vi "BRig_RT__Case_Exp__State_initTrial__LC_Cue__v18.vi"(6 "input_arrTrig":bool[](array[boolean]), 8 "input_dataTrial":u16[][](array[numeric]), 9 "input_dataExp":u16[](array[numeric]), 10 "input_dataLC":u16[](array[numeric]), 11 "input_dataCurrent":u16[](array[numeric])) -> (0 "output_dataTrial":u16[][](array[numeric]), 3 "output_dataCurrent":u16[](array[numeric]), 4 "output_arrTrig":bool[](array[boolean]))   [LabVIEW 2014]
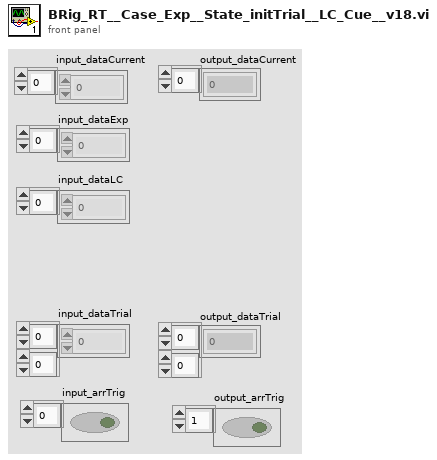
[diagram p1: front panel]
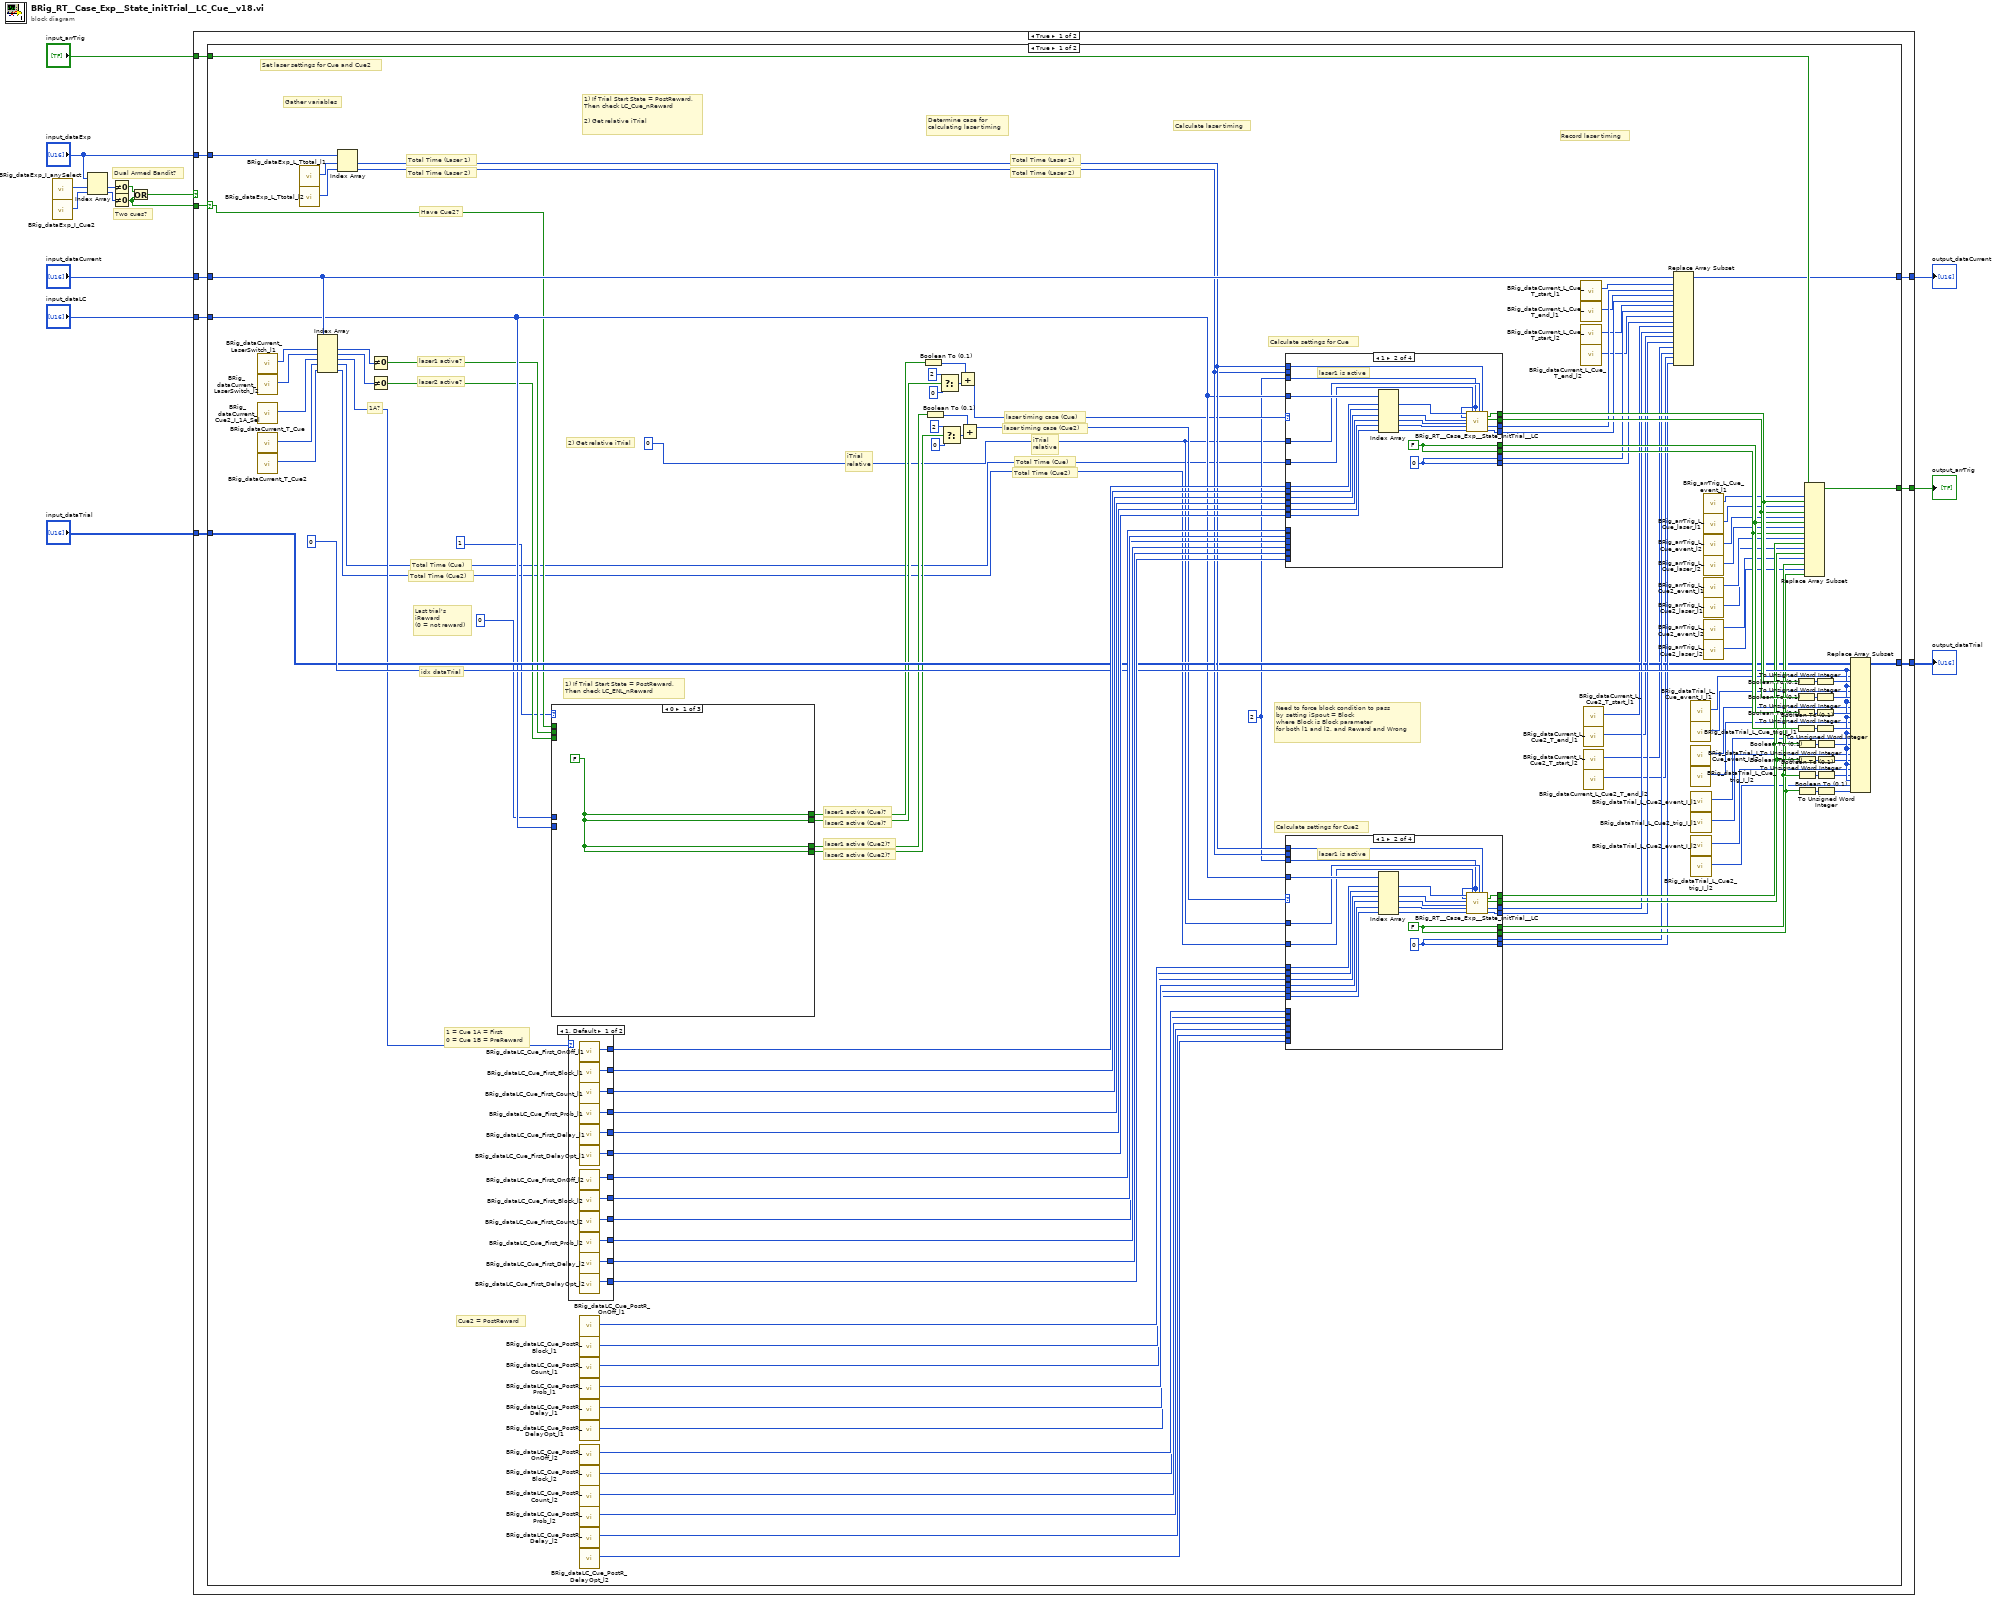
[diagram p0: block diagram]
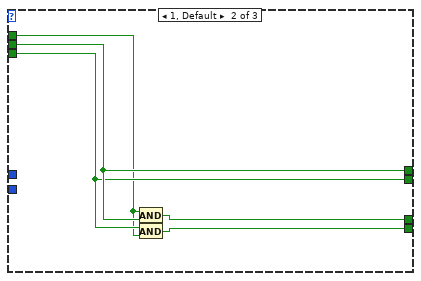
[diagram p2: hidden frame]
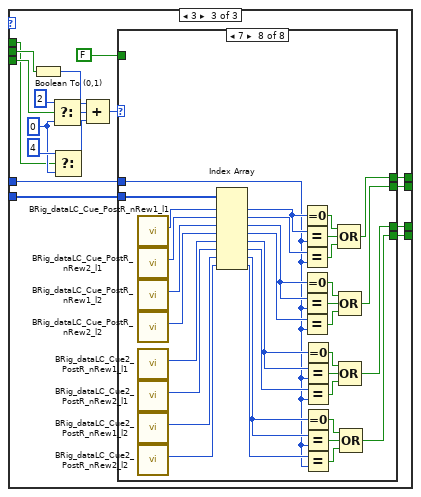
[diagram p3: hidden frame]
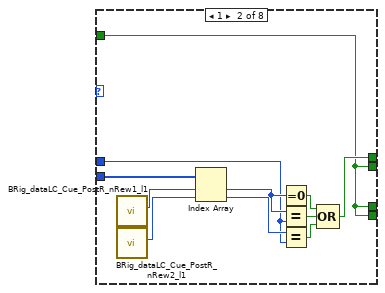
[diagram p5: hidden frame]
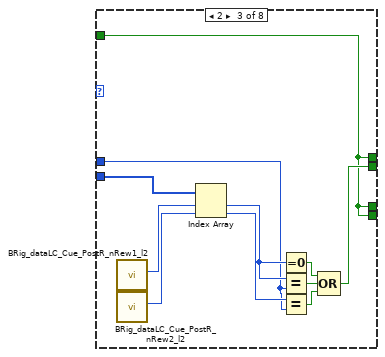
[diagram p6: hidden frame]
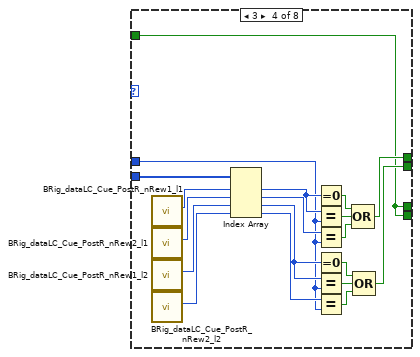
[diagram p7: hidden frame]
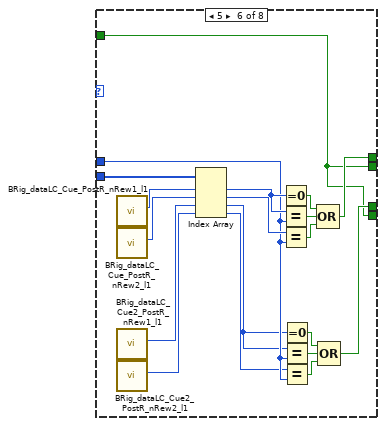
[diagram p9: hidden frame]
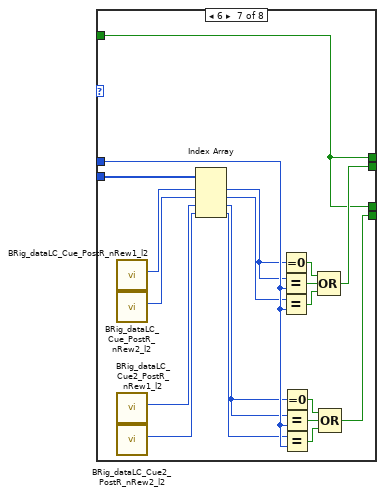
[diagram p10: hidden frame]
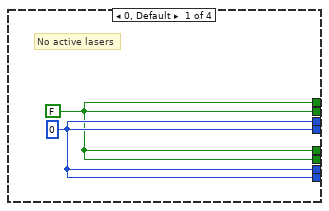
[diagram p11: hidden frame]
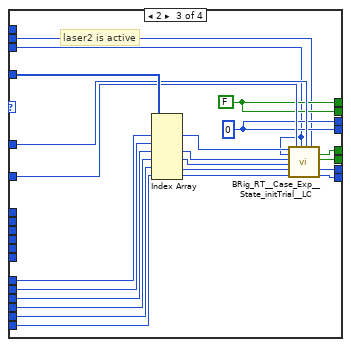
[diagram p12: hidden frame]
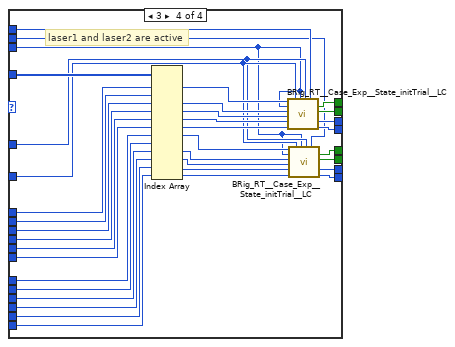
[diagram p13: hidden frame]
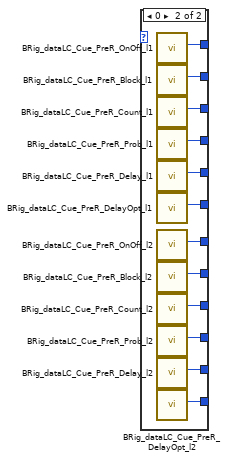
[diagram p14: hidden frame]
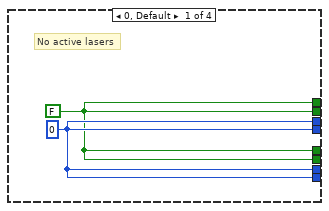
[diagram p15: hidden frame]
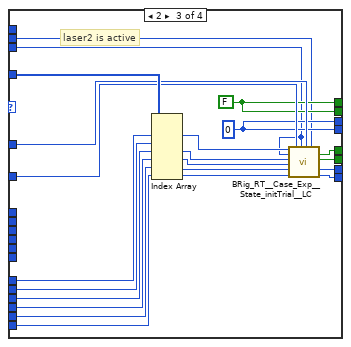
[diagram p16: hidden frame]
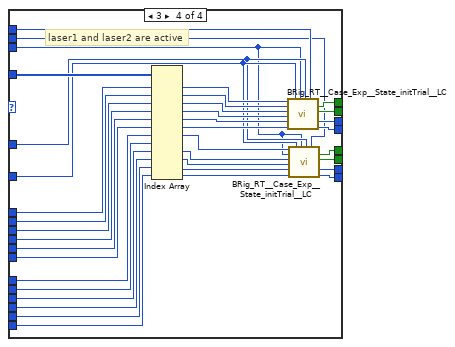
[diagram p17: hidden frame]
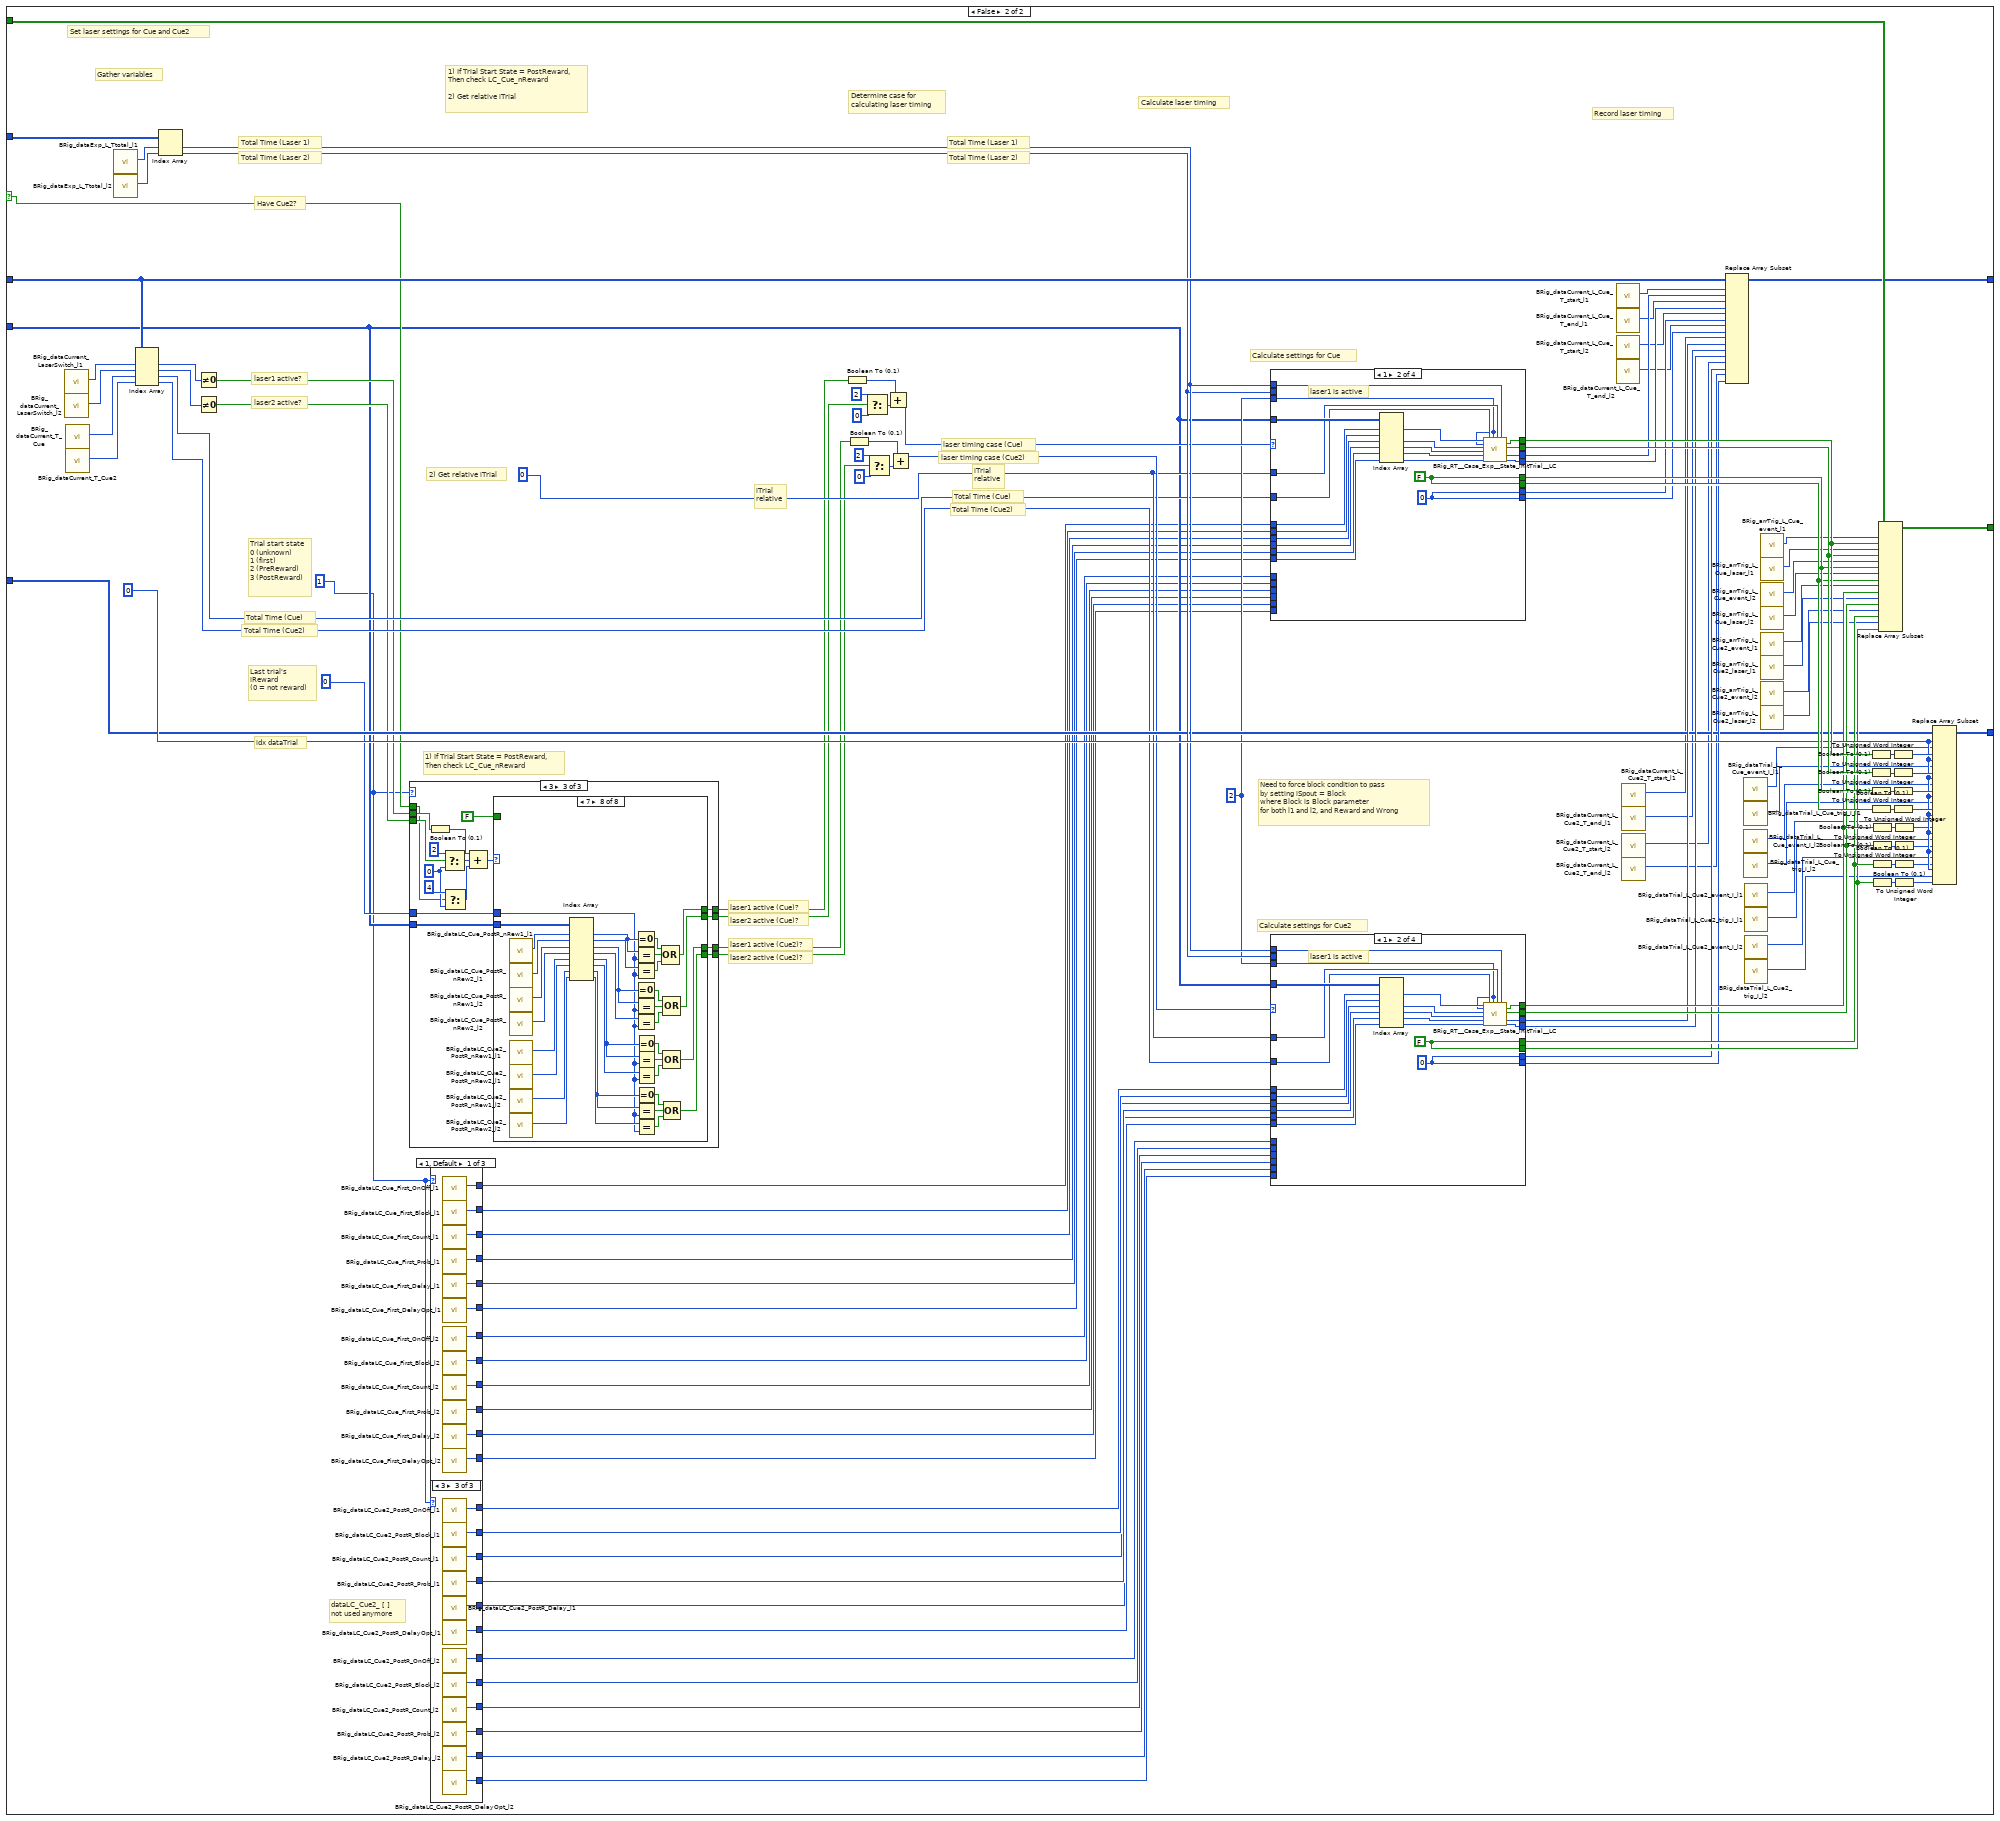
[diagram p18: hidden frame]
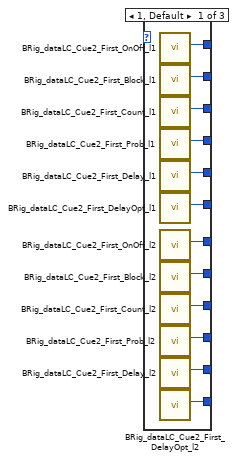
[diagram p19: hidden frame]
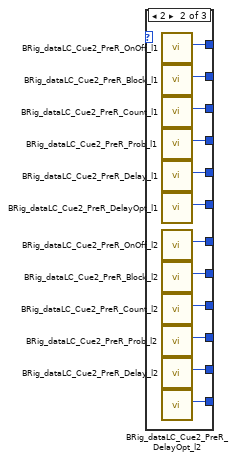
[diagram p20: hidden frame]
diagram:
  # "Two cues?"
  # "Dual Armed Bandit?"
  n1 = call "BRig_dataExp_I_anySelect.vi"() -> ("output_I_anySelect"=w8:i32)  [unwired: 11 in]
  n2 = call "BRig_dataExp_I_Cue2.vi"() -> ("output_I_Cue2"=w6:i32)  [unwired: 11 in]
  n3 = Index Array(array="input_dataExp", index #1=w8, index #2=w6) -> (element #1=w7:u16, element #2=w5:u16)
  n4 = Not Equal To 0?(x=w7) -> (x != 0?=w4:bool)
  n5 = Not Equal To 0?(x=w5) -> (x != 0?=w1:bool)
  n6 = Or(x=w4, y=w1) -> (x .or. y?=w2:bool)
  n7 = case shown="True" w2 {
    tunnel: "input_arrTrig" -> [w24 w1044]
    tunnel: [w23 w1043] -> w14
    tunnel: [w22 w1030] -> w13
    tunnel: "input_dataCurrent" -> [w21 w1029]
    tunnel: [w20 w1028] -> w11
    tunnel: "input_dataExp" -> [w19 w1021]
    tunnel: "input_dataTrial" -> [w18 w1012]
    tunnel: "input_dataLC" -> [w17 w1000]
    tunnel: w1 -> [w16 _]
    frame True {
      n8 = case shown="True" w16 {
        selector: w16 -> [w69 w533]
        tunnel: w24 -> [w140 w589]
        tunnel: [w139 w588] -> w23
        tunnel: [w126 w575] -> w22
        tunnel: w21 -> [w125 w574]
        tunnel: [w124 w573] -> w20
        tunnel: w19 -> [w105 w566]
        tunnel: w18 -> [w85 w546]
        tunnel: w17 -> [w84 w529]
        frame True {
          w70 = u16 0
          w71 = u16 2 ("input_sState_start")
          w100 = 0
          # "Cue2 = PostReward"
          # "1 = Cue 1A = First\n0 = Cue 1B = PreReward"
          # "1A?"
          # "Need to force block condition to pass\nby setting iSpout = Block\nwhere Block is Block parameter\nfor both l1 and l2, and Reward and Wrong"
          # "Record laser timing"
          # "Calculate laser timing"
          # "Total Time (Cue2)"
          # "Total Time (Cue)"
          # "iTrial\nrelative"
          # "Total Time (Laser 2)"
          # "Total Time (Laser 1)"
          # "laser timing case (Cue2)"
          # "Determine case for\ncalculating laser timing"
          # "2) Get relative iTrial"
          # "1) If Trial Start State = PostReward,\nThen check LC_ENL_nReward"
          # "laser2 active (Cue2)?"
          # "laser1 active (Cue2)?"
          # "laser2 active (Cue)?"
          # "laser1 active (Cue)?"
          # "1) If Trial Start State = PostReward,\nThen check LC_Cue_nReward\n\n2) Get relative iTrial"
          # "Gather variables"
          # "Last trial's\niReward\n(0 = not reward)"
          # "idx dataTrial"
          # "Total Time (Cue2)"
          # "Total Time (Cue)"
          # "Have Cue2?"
          # "Total Time (Laser 2)"
          # "Total Time (Laser 1)"
          # "Calculate settings for Cue2"
          # "Calculate settings for Cue"
          # "Set laser settings for Cue and Cue2"
          # "iTrial\nrelative"
          # "laser timing case (Cue)"
          # "laser2 active?"
          # "laser1 active?"
          n9 = call "BRig_dataCurrent_LaserSwitch_l1.vi"() -> ("output_LaserSwitch_l1"=w148:i32)  [unwired: 11 in]
          n10 = call "BRig_dataCurrent_LaserSwitch_l2.vi"() -> ("output_LaserSwitch_l2"=w147:i32)  [unwired: 11 in]
          n11 = call "BRig_dataCurrent_Cue2_I_1A_Sel.vi"() -> ("output_Cue2_I_1A_Sel"=w67:i32)  [unwired: 11 in]
          n12 = call "BRig_dataCurrent_T_Cue.vi"() -> ("output_T_Cue"=w64:i32)  [unwired: 11 in]
          n13 = call "BRig_dataCurrent_T_Cue2.vi"() -> ("output_T_Cue2"=w63:i32)  [unwired: 11 in]
          n14 = call "BRig_dataExp_L_Ttotal_l1.vi"() -> ("output_L_Ttotal_l1"=w106:i32)  [unwired: 11 in]
          n15 = call "BRig_dataExp_L_Ttotal_l2.vi"() -> ("output_L_Ttotal_l2"=w107:i32)  [unwired: 11 in]
          n16 = Index Array(array=w125, index #1=w148, index #2=w147, index #3=w67, index #4=w64, index #5=w63) -> (element #1=w146:u16, element #2=w145:u16, element #3=w66:u16, element #4=w61:u16, element #5=w62:u16)
          n17 = Index Array(array=w105, index #1=w106, index #2=w107) -> (element #1=w95:u16, element #2=w94:u16)
          n18 = Not Equal To 0?(x=w146) -> (x != 0?=w82:bool)
          n19 = Not Equal To 0?(x=w145) -> (x != 0?=w83:bool)
          n20 = case shown="0" u16 1 {
            tunnel: u16 0 -> [_ _ w162]
            tunnel: w84 -> [_ _ w161]
            tunnel: w83 -> [_ w153 w164]
            tunnel: w82 -> [_ w154 w165]
            tunnel: w69 -> [_ w152 w163]
            tunnel: [w149 w154 w158] -> w81
            tunnel: [w149 w153 w157] -> w80
            tunnel: [w149 w151 w156] -> w75
            tunnel: [w149 w150 w155] -> w74
            frame 0 {
              w149 = FALSE
            }
            frame 1, Default {
              n21 = And(x=w152, y=w154) -> (x .and. y?=w151:bool)
              n22 = And(x=w153, y=w152) -> (x .and. y?=w150:bool)
            }
            frame 3 {
              w169 = i16 0 ("f")
              n23 = Boolean To (0,1)(Boolean=w165) -> (0, 1=w167:i16)
              n24 = Select(t=i16 2, s=w164, f=w169) -> (s? t:f=w168:i16)
              n25 = Select(t=i16 4, s=w163, f=w169) -> (s? t:f=w166:i16)
              n26 = Compound Arithmetic op=ADD(w167, w168, w166) -> (w159:i16)
              n27 = case shown="7" w159 {
                tunnel: w161 -> [_ w178 w189 w203 _ w228 w249 w276]
                tunnel: w162 -> [_ w177 w188 w202 _ w224 w245 w265]
                tunnel: [w172 w176 w186 w201 w214 w223 w242 w264] -> w158
                tunnel: [w172 w175 w187 w200 w214 w221 w244 w263] -> w157
                tunnel: [w172 w175 w186 w199 w214 w222 w242 w262] -> w156
                tunnel: [w172 w175 w186 w199 w214 w221 w243 w261] -> w155
                tunnel: FALSE -> [w172 w175 w186 w199 w214 w221 w242 _]
                frame 0, Default {
                }
                frame 1 {
                  n28 = call "BRig_dataLC_Cue_PostR_nRew1_l1.vi"() -> ("output_Cue_PostR_nRew1_l1"=w173:i32)  [unwired: 11 in]
                  n29 = call "BRig_dataLC_Cue_PostR_nRew2_l1.vi"() -> ("output_Cue_PostR_nRew2_l1"=w174:i32)  [unwired: 11 in]
                  n30 = Index Array(array=w178, index #1=w173, index #2=w174) -> (element #1=w180:u16, element #2=w179:u16)
                  n31 = Equal To 0?(x=w180) -> (x = 0?=w181:bool)
                  n32 = Equal?(x=w180, y=w177) -> (x = y?=w182:bool)
                  n33 = Equal?(x=w179, y=w177) -> (x = y?=w183:bool)
                  n34 = Compound Arithmetic op=OR(w181, w182, w183) -> (w176:bool)
                }
                frame 2 {
                  n35 = call "BRig_dataLC_Cue_PostR_nRew1_l2.vi"() -> ("output_Cue_PostR_nRew1_l2"=w184:i32)  [unwired: 11 in]
                  n36 = call "BRig_dataLC_Cue_PostR_nRew2_l2.vi"() -> ("output_Cue_PostR_nRew2_l2"=w185:i32)  [unwired: 11 in]
                  n37 = Index Array(array=w189, index #1=w184, index #2=w185) -> (element #1=w190:u16, element #2=w191:u16)
                  n38 = Equal To 0?(x=w190) -> (x = 0?=w193:bool)
                  n39 = Equal?(x=w190, y=w188) -> (x = y?=w192:bool)
                  n40 = Equal?(x=w191, y=w188) -> (x = y?=w194:bool)
                  n41 = Compound Arithmetic op=OR(w193, w192, w194) -> (w187:bool)
                }
                frame 3 {
                  n42 = call "BRig_dataLC_Cue_PostR_nRew1_l1.vi"() -> ("output_Cue_PostR_nRew1_l1"=w195:i32)  [unwired: 11 in]
                  n43 = call "BRig_dataLC_Cue_PostR_nRew2_l1.vi"() -> ("output_Cue_PostR_nRew2_l1"=w196:i32)  [unwired: 11 in]
                  n44 = call "BRig_dataLC_Cue_PostR_nRew1_l2.vi"() -> ("output_Cue_PostR_nRew1_l2"=w197:i32)  [unwired: 11 in]
                  n45 = call "BRig_dataLC_Cue_PostR_nRew2_l2.vi"() -> ("output_Cue_PostR_nRew2_l2"=w198:i32)  [unwired: 11 in]
                  n46 = Index Array(array=w203, index #1=w195, index #2=w196, index #3=w197, index #4=w198) -> (element #1=w207:u16, element #2=w206:u16, element #3=w204:u16, element #4=w205:u16)
                  n47 = Equal To 0?(x=w207) -> (x = 0?=w208:bool)
                  n48 = Equal?(x=w207, y=w202) -> (x = y?=w209:bool)
                  n49 = Equal?(x=w206, y=w202) -> (x = y?=w210:bool)
                  n50 = Equal To 0?(x=w204) -> (x = 0?=w212:bool)
                  n51 = Equal?(x=w204, y=w202) -> (x = y?=w211:bool)
                  n52 = Equal?(x=w205, y=w202) -> (x = y?=w213:bool)
                  n53 = Compound Arithmetic op=OR(w208, w209, w210) -> (w201:bool)
                  n54 = Compound Arithmetic op=OR(w212, w211, w213) -> (w200:bool)
                }
                frame 4 {
                }
                frame 5 {
                  n55 = call "BRig_dataLC_Cue_PostR_nRew1_l1.vi"() -> ("output_Cue_PostR_nRew1_l1"=w217:i32)  [unwired: 11 in]
                  n56 = call "BRig_dataLC_Cue_PostR_nRew2_l1.vi"() -> ("output_Cue_PostR_nRew2_l1"=w218:i32)  [unwired: 11 in]
                  n57 = call "BRig_dataLC_Cue2_PostR_nRew1_l1.vi"() -> ("output_Cue2_PostR_nRew1_l1"=w215:i32)  [unwired: 11 in]
                  n58 = call "BRig_dataLC_Cue2_PostR_nRew2_l1.vi"() -> ("output_Cue2_PostR_nRew2_l1"=w216:i32)  [unwired: 11 in]
                  n59 = Index Array(array=w228, index #1=w217, index #2=w218, index #3=w215, index #4=w216) -> (element #1=w230:u16, element #2=w229:u16, element #3=w220:u16, element #4=w219:u16)
                  n60 = Equal To 0?(x=w230) -> (x = 0?=w231:bool)
                  n61 = Equal?(x=w230, y=w224) -> (x = y?=w232:bool)
                  n62 = Equal?(x=w229, y=w224) -> (x = y?=w233:bool)
                  n63 = Equal To 0?(x=w220) -> (x = 0?=w227:bool)
                  n64 = Equal?(x=w220, y=w224) -> (x = y?=w226:bool)
                  n65 = Equal?(x=w219, y=w224) -> (x = y?=w225:bool)
                  n66 = Compound Arithmetic op=OR(w231, w232, w233) -> (w223:bool)
                  n67 = Compound Arithmetic op=OR(w227, w226, w225) -> (w222:bool)
                }
                frame 6 {
                  n68 = call "BRig_dataLC_Cue_PostR_nRew1_l2.vi"() -> ("output_Cue_PostR_nRew1_l2"=w237:i32)  [unwired: 11 in]
                  n69 = call "BRig_dataLC_Cue_PostR_nRew2_l2.vi"() -> ("output_Cue_PostR_nRew2_l2"=w236:i32)  [unwired: 11 in]
                  n70 = call "BRig_dataLC_Cue2_PostR_nRew1_l2.vi"() -> ("output_Cue2_PostR_nRew1_l2"=w235:i32)  [unwired: 11 in]
                  n71 = call "BRig_dataLC_Cue2_PostR_nRew2_l2.vi"() -> ("output_Cue2_PostR_nRew2_l2"=w234:i32)  [unwired: 11 in]
                  n72 = Index Array(array=w249, index #1=w237, index #2=w236, index #3=w235, index #4=w234) -> (element #1=w241:u16, element #2=w240:u16, element #3=w239:u16, element #4=w238:u16)
                  n73 = Equal To 0?(x=w241) -> (x = 0?=w251:bool)
                  n74 = Equal?(x=w241, y=w245) -> (x = y?=w250:bool)
                  n75 = Equal?(x=w240, y=w245) -> (x = y?=w252:bool)
                  n76 = Equal To 0?(x=w239) -> (x = 0?=w247:bool)
                  n77 = Equal?(x=w239, y=w245) -> (x = y?=w248:bool)
                  n78 = Equal?(x=w238, y=w245) -> (x = y?=w246:bool)
                  n79 = Compound Arithmetic op=OR(w251, w250, w252) -> (w244:bool)
                  n80 = Compound Arithmetic op=OR(w247, w248, w246) -> (w243:bool)
                }
                frame 7 {
                  n81 = call "BRig_dataLC_Cue_PostR_nRew1_l1.vi"() -> ("output_Cue_PostR_nRew1_l1"=w257:i32)  [unwired: 11 in]
                  n82 = call "BRig_dataLC_Cue_PostR_nRew2_l1.vi"() -> ("output_Cue_PostR_nRew2_l1"=w258:i32)  [unwired: 11 in]
                  n83 = call "BRig_dataLC_Cue_PostR_nRew1_l2.vi"() -> ("output_Cue_PostR_nRew1_l2"=w259:i32)  [unwired: 11 in]
                  n84 = call "BRig_dataLC_Cue_PostR_nRew2_l2.vi"() -> ("output_Cue_PostR_nRew2_l2"=w260:i32)  [unwired: 11 in]
                  n85 = call "BRig_dataLC_Cue2_PostR_nRew1_l1.vi"() -> ("output_Cue2_PostR_nRew1_l1"=w256:i32)  [unwired: 11 in]
                  n86 = call "BRig_dataLC_Cue2_PostR_nRew2_l1.vi"() -> ("output_Cue2_PostR_nRew2_l1"=w255:i32)  [unwired: 11 in]
                  n87 = call "BRig_dataLC_Cue2_PostR_nRew1_l2.vi"() -> ("output_Cue2_PostR_nRew1_l2"=w254:i32)  [unwired: 11 in]
                  n88 = call "BRig_dataLC_Cue2_PostR_nRew2_l2.vi"() -> ("output_Cue2_PostR_nRew2_l2"=w253:i32)  [unwired: 11 in]
                  n89 = Index Array(array=w276, index #1=w257, index #2=w258, index #3=w259, index #4=w260, index #5=w256, index #6=w255, index #7=w254, index #8=w253) -> (element #1=w280:u16, element #2=w279:u16, element #3=w277:u16, element #4=w278:u16, element #5=w269:u16, element #6=w268:u16, element #7=w266:u16, element #8=w267:u16)
                  n90 = Equal To 0?(x=w280) -> (x = 0?=w281:bool)
                  n91 = Equal?(x=w280, y=w265) -> (x = y?=w282:bool)
                  n92 = Equal?(x=w279, y=w265) -> (x = y?=w283:bool)
                  n93 = Equal To 0?(x=w277) -> (x = 0?=w285:bool)
                  n94 = Equal?(x=w277, y=w265) -> (x = y?=w284:bool)
                  n95 = Equal?(x=w278, y=w265) -> (x = y?=w286:bool)
                  n96 = Equal To 0?(x=w269) -> (x = 0?=w275:bool)
                  n97 = Equal?(x=w269, y=w265) -> (x = y?=w274:bool)
                  n98 = Equal?(x=w268, y=w265) -> (x = y?=w273:bool)
                  n99 = Equal To 0?(x=w266) -> (x = 0?=w271:bool)
                  n100 = Equal?(x=w266, y=w265) -> (x = y?=w272:bool)
                  n101 = Equal?(x=w267, y=w265) -> (x = y?=w270:bool)
                  n102 = Compound Arithmetic op=OR(w281, w282, w283) -> (w264:bool)
                  n103 = Compound Arithmetic op=OR(w285, w284, w286) -> (w263:bool)
                  n104 = Compound Arithmetic op=OR(w275, w274, w273) -> (w262:bool)
                  n105 = Compound Arithmetic op=OR(w271, w272, w270) -> (w261:bool)
                }
              }
            }
          }
          n106 = case shown="1, Default" w66 {
            tunnel: [w370 w382] -> w119
            tunnel: [w371 w383] -> w118
            tunnel: [w372 w384] -> w117
            tunnel: [w373 w385] -> w116
            tunnel: [w374 w386] -> w115
            tunnel: [w375 w387] -> w114
            tunnel: [w376 w388] -> w113
            tunnel: [w377 w389] -> w112
            tunnel: [w378 w390] -> w111
            tunnel: [w379 w391] -> w110
            tunnel: [w380 w392] -> w109
            tunnel: [w369 w381] -> w108
            frame 1, Default {
              n107 = call "BRig_dataLC_Cue_First_OnOff_l1.vi"() -> ("output_Cue_First_OnOff"=w370:i32)  [unwired: 11 in]
              n108 = call "BRig_dataLC_Cue_First_Block_l1.vi"() -> ("output_Cue_First_Block"=w371:i32)  [unwired: 11 in]
              n109 = call "BRig_dataLC_Cue_First_Count_l1.vi"() -> ("output_Cue_First_Count"=w372:i32)  [unwired: 11 in]
              n110 = call "BRig_dataLC_Cue_First_Prob_l1.vi"() -> ("output_Cue_First_Prob"=w373:i32)  [unwired: 11 in]
              n111 = call "BRig_dataLC_Cue_First_Delay_l1.vi"() -> ("output_Cue_First_Delay"=w374:i32)  [unwired: 11 in]
              n112 = call "BRig_dataLC_Cue_First_DelayOpt_l1.vi"() -> ("output_Cue_First_DelayOpt"=w375:i32)  [unwired: 11 in]
              n113 = call "BRig_dataLC_Cue_First_OnOff_l2.vi"() -> ("output_Cue_First_OnOff_l2"=w376:i32)  [unwired: 11 in]
              n114 = call "BRig_dataLC_Cue_First_Block_l2.vi"() -> ("output_Cue_First_Block_l2"=w377:i32)  [unwired: 11 in]
              n115 = call "BRig_dataLC_Cue_First_Count_l2.vi"() -> ("output_Cue_First_Count_l2"=w378:i32)  [unwired: 11 in]
              n116 = call "BRig_dataLC_Cue_First_Prob_l2.vi"() -> ("output_Cue_First_Prob_l2"=w379:i32)  [unwired: 11 in]
              n117 = call "BRig_dataLC_Cue_First_Delay_l2.vi"() -> ("output_Cue_First_Delay_l2"=w380:i32)  [unwired: 11 in]
              n118 = call "BRig_dataLC_Cue_First_DelayOpt_l2.vi"() -> ("output_Cue_First_DelayOpt_l2"=w369:i32)  [unwired: 11 in]
            }
            frame 0 {
              n119 = call "BRig_dataLC_Cue_PreR_OnOff_l1.vi"() -> ("output_Cue_PreR_OnOff"=w382:i32)  [unwired: 11 in]
              n120 = call "BRig_dataLC_Cue_PreR_Block_l1.vi"() -> ("output_Cue_PreR_Block"=w383:i32)  [unwired: 11 in]
              n121 = call "BRig_dataLC_Cue_PreR_Count_l1.vi"() -> ("output_Cue_PreR_Count"=w384:i32)  [unwired: 11 in]
              n122 = call "BRig_dataLC_Cue_PreR_Prob_l1.vi"() -> ("output_Cue_PreR_Prob"=w385:i32)  [unwired: 11 in]
              n123 = call "BRig_dataLC_Cue_PreR_Delay_l1.vi"() -> ("output_Cue_PreR_Delay"=w386:i32)  [unwired: 11 in]
              n124 = call "BRig_dataLC_Cue_PreR_DelayOpt_l1.vi"() -> ("output_Cue_PreR_DelayOpt"=w387:i32)  [unwired: 11 in]
              n125 = call "BRig_dataLC_Cue_PreR_OnOff_l2.vi"() -> ("output_Cue_PreR_OnOff_l2"=w388:i32)  [unwired: 11 in]
              n126 = call "BRig_dataLC_Cue_PreR_Block_l2.vi"() -> ("output_Cue_PreR_Block_l2"=w389:i32)  [unwired: 11 in]
              n127 = call "BRig_dataLC_Cue_PreR_Count_l2.vi"() -> ("output_Cue_PreR_Count_l2"=w390:i32)  [unwired: 11 in]
              n128 = call "BRig_dataLC_Cue_PreR_Prob_l2.vi"() -> ("output_Cue_PreR_Prob_l2"=w391:i32)  [unwired: 11 in]
              n129 = call "BRig_dataLC_Cue_PreR_Delay_l2.vi"() -> ("output_Cue_PreR_Delay_l2"=w392:i32)  [unwired: 11 in]
              n130 = call "BRig_dataLC_Cue_PreR_DelayOpt_l2.vi"() -> ("output_Cue_PreR_DelayOpt_l2"=w381:i32)  [unwired: 11 in]
            }
          }
          n131 = call "BRig_dataLC_Cue_PostR_OnOff_l1.vi"() -> ("output_Cue_PostR_OnOff"=w60:i32)  [unwired: 11 in]
          n132 = call "BRig_dataLC_Cue_PostR_Block_l1.vi"() -> ("output_Cue_PostR_Block"=w59:i32)  [unwired: 11 in]
          n133 = call "BRig_dataLC_Cue_PostR_Count_l1.vi"() -> ("output_Cue_PostR_Count"=w58:i32)  [unwired: 11 in]
          n134 = call "BRig_dataLC_Cue_PostR_Prob_l1.vi"() -> ("output_Cue_PostR_Prob"=w57:i32)  [unwired: 11 in]
          n135 = call "BRig_dataLC_Cue_PostR_Delay_l1.vi"() -> ("output_Cue_PostR_Delay"=w56:i32)  [unwired: 11 in]
          n136 = call "BRig_dataLC_Cue_PostR_DelayOpt_l1.vi"() -> ("output_Cue_PostR_DelayOpt"=w55:i32)  [unwired: 11 in]
          n137 = call "BRig_dataLC_Cue_PostR_OnOff_l2.vi"() -> ("output_Cue_PostR_OnOff_l2"=w54:i32)  [unwired: 11 in]
          n138 = call "BRig_dataLC_Cue_PostR_Block_l2.vi"() -> ("output_Cue_PostR_Block_l2"=w53:i32)  [unwired: 11 in]
          n139 = call "BRig_dataLC_Cue_PostR_Count_l2.vi"() -> ("output_Cue_PostR_Count_l2"=w52:i32)  [unwired: 11 in]
          n140 = call "BRig_dataLC_Cue_PostR_Prob_l2.vi"() -> ("output_Cue_PostR_Prob_l2"=w51:i32)  [unwired: 11 in]
          n141 = call "BRig_dataLC_Cue_PostR_Delay_l2.vi"() -> ("output_Cue_PostR_Delay_l2"=w50:i32)  [unwired: 11 in]
          n142 = call "BRig_dataLC_Cue_PostR_DelayOpt_l2.vi"() -> ("output_Cue_PostR_DelayOpt_l2"=w49:i32)  [unwired: 11 in]
          n143 = Boolean To (0,1)(Boolean=w81) -> (0, 1=w142:i16)
          n144 = Boolean To (0,1)(Boolean=w75) -> (0, 1=w78:i16)
          n145 = Select(t=i16 2, s=w80, f=i16 0) -> (s? t:f=w143:i16)
          n146 = Select(t=i16 2, s=w74, f=i16 0) -> (s? t:f=w77:i16)
          n147 = Add(x=w142, y=w143) -> (x+y=w73:i16)
          n148 = Add(x=w78, y=w77) -> (x+y=w72:i16)
          n149 = case shown="1" w73 {
            tunnel: w84 -> [_ w416 w438 w475]
            tunnel: w71 -> [_ w395 w417 w439]
            tunnel: w61 -> [_ w410 w432 w463]
            tunnel: w70 -> [_ w409 w431 w462]
            tunnel: [w393 w408 w420 w461] -> w134
            tunnel: [w393 w407 w420 w460] -> w131
            tunnel: [w394 w406 w419 w459] -> w123
            tunnel: [w394 w405 w419 w458] -> w122
            tunnel: [w393 w398 w430 w457] -> w127
            tunnel: [w394 w397 w429 w456] -> w121
            tunnel: [w393 w398 w428 w455] -> w129
            tunnel: [w394 w397 w427 w454] -> w120
            tunnel: w119 -> [_ w404 _ w453]
            tunnel: w118 -> [_ w403 _ w452]
            tunnel: w117 -> [_ w402 _ w451]
            tunnel: w116 -> [_ w401 _ w450]
            tunnel: w115 -> [_ w400 _ w449]
            tunnel: w114 -> [_ w399 _ w448]
            tunnel: w113 -> [_ _ w426 w447]
            tunnel: w112 -> [_ _ w425 w446]
            tunnel: w111 -> [_ _ w424 w445]
            tunnel: w110 -> [_ _ w423 w444]
            tunnel: w109 -> [_ _ w422 w443]
            tunnel: w108 -> [_ _ w421 w442]
            tunnel: w95 -> [_ w396 _ w441]
            tunnel: w94 -> [_ _ w418 w440]
            frame 0, Default {
              w394 = u16 0
              w393 = FALSE
              # "No active lasers"
            }
            frame 1 {
              w397 = u16 0
              w398 = FALSE
              # "laser1 is active"
              n150 = Index Array(array=w416, index #1=w404, index #2=w403, index #3=w402, index #4=w401, index #5=w400, index #6=w399) -> (element #1=w415:u16, element #3=w414:u16, element #4=w413:u16, element #5=w412:u16, element #6=w411:u16)  [unwired: 1 out]
              n151 = call "BRig_RT__Case_Exp__State_initTrial__LC.vi"("input_L_OnOff"=w415, "input_L_Block"=w395, "input_L_Count"=w414, "input_L_Prob"=w413, "input_L_Tdelay"=w412, "input_L_delayOpt"=w411, "input_T_state"=w410, "input_iSpout"=w395, "input_iTrial_relative"=w409, "input_L_T"=w396) -> ("output_LC_Event"=w408:bool, "output_LC_Laser"=w407:bool, "output_L_Tstart"=w406:u16, "output_L_Tend"=w405:u16)  [unwired: 6 in]
            }
            frame 2 {
              w419 = u16 0
              w420 = FALSE
              # "laser2 is active"
              n152 = Index Array(array=w438, index #1=w426, index #2=w425, index #3=w424, index #4=w423, index #5=w422, index #6=w421) -> (element #1=w433:u16, element #3=w434:u16, element #4=w435:u16, element #5=w436:u16, element #6=w437:u16)  [unwired: 1 out]
              n153 = call "BRig_RT__Case_Exp__State_initTrial__LC.vi"("input_L_OnOff"=w433, "input_L_Block"=w417, "input_L_Count"=w434, "input_L_Prob"=w435, "input_L_Tdelay"=w436, "input_L_delayOpt"=w437, "input_T_state"=w432, "input_iSpout"=w417, "input_iTrial_relative"=w431, "input_L_T"=w418) -> ("output_LC_Event"=w428:bool, "output_LC_Laser"=w430:bool, "output_L_Tstart"=w429:u16, "output_L_Tend"=w427:u16)  [unwired: 6 in]
            }
            frame 3 {
              # "laser1 and laser2 are active"
              n154 = Index Array(array=w475, index #1=w453, index #2=w452, index #3=w451, index #4=w450, index #5=w449, index #6=w448, index #7=w447, index #8=w446, index #9=w445, index #10=w444, index #11=w443, index #12=w442) -> (element #1=w474:u16, element #2=w473:u16, element #3=w472:u16, element #4=w471:u16, element #5=w470:u16, element #6=w469:u16, element #7=w464:u16, element #9=w465:u16, element #10=w466:u16, element #11=w467:u16, element #12=w468:u16)  [unwired: 1 out]
              n155 = call "BRig_RT__Case_Exp__State_initTrial__LC.vi"("input_L_OnOff"=w474, "input_L_Block"=w473, "input_L_Count"=w472, "input_L_Prob"=w471, "input_L_Tdelay"=w470, "input_L_delayOpt"=w469, "input_T_state"=w463, "input_iSpout"=w439, "input_iTrial_relative"=w462, "input_L_T"=w441) -> ("output_LC_Event"=w461:bool, "output_LC_Laser"=w460:bool, "output_L_Tstart"=w459:u16, "output_L_Tend"=w458:u16)  [unwired: 6 in]
              n156 = call "BRig_RT__Case_Exp__State_initTrial__LC.vi"("input_L_OnOff"=w464, "input_L_Block"=w439, "input_L_Count"=w465, "input_L_Prob"=w466, "input_L_Tdelay"=w467, "input_L_delayOpt"=w468, "input_T_state"=w463, "input_iSpout"=w439, "input_iTrial_relative"=w462, "input_L_T"=w440) -> ("output_LC_Event"=w455:bool, "output_LC_Laser"=w457:bool, "output_L_Tstart"=w456:u16, "output_L_Tend"=w454:u16)  [unwired: 6 in]
            }
          }
          n157 = case shown="1" w72 {
            tunnel: w84 -> [_ w310 w332 w368]
            tunnel: w71 -> [_ w289 w311 w333]
            tunnel: w62 -> [_ w304 w326 w357]
            tunnel: w70 -> [_ w303 w325 w356]
            tunnel: [w287 w302 w314 w355] -> w93
            tunnel: [w287 w301 w314 w354] -> w92
            tunnel: [w288 w300 w313 w353] -> w89
            tunnel: [w288 w299 w313 w352] -> w88
            tunnel: [w287 w292 w324 w351] -> w90
            tunnel: [w288 w291 w323 w350] -> w87
            tunnel: [w287 w292 w322 w349] -> w91
            tunnel: [w288 w291 w321 w348] -> w86
            tunnel: w60 -> [_ w298 _ w347]
            tunnel: w59 -> [_ w297 _ w346]
            tunnel: w58 -> [_ w296 _ w345]
            tunnel: w57 -> [_ w295 _ w344]
            tunnel: w56 -> [_ w294 _ w343]
            tunnel: w55 -> [_ w293 _ w342]
            tunnel: w54 -> [_ _ w320 w341]
            tunnel: w53 -> [_ _ w319 w340]
            tunnel: w52 -> [_ _ w318 w339]
            tunnel: w51 -> [_ _ w317 w338]
            tunnel: w50 -> [_ _ w316 w337]
            tunnel: w49 -> [_ _ w315 w336]
            tunnel: w95 -> [_ w290 _ w335]
            tunnel: w94 -> [_ _ w312 w334]
            frame 0, Default {
              w288 = u16 0
              w287 = FALSE
              # "No active lasers"
            }
            frame 1 {
              w291 = u16 0
              w292 = FALSE
              # "laser1 is active"
              n158 = Index Array(array=w310, index #1=w298, index #2=w297, index #3=w296, index #4=w295, index #5=w294, index #6=w293) -> (element #1=w309:u16, element #3=w308:u16, element #4=w307:u16, element #5=w306:u16, element #6=w305:u16)  [unwired: 1 out]
              n159 = call "BRig_RT__Case_Exp__State_initTrial__LC.vi"("input_L_OnOff"=w309, "input_L_Block"=w289, "input_L_Count"=w308, "input_L_Prob"=w307, "input_L_Tdelay"=w306, "input_L_delayOpt"=w305, "input_T_state"=w304, "input_iSpout"=w289, "input_iTrial_relative"=w303, "input_L_T"=w290) -> ("output_LC_Event"=w302:bool, "output_LC_Laser"=w301:bool, "output_L_Tstart"=w300:u16, "output_L_Tend"=w299:u16)  [unwired: 6 in]
            }
            frame 2 {
              w313 = u16 0
              w314 = FALSE
              # "laser2 is active"
              n160 = Index Array(array=w332, index #1=w320, index #2=w319, index #3=w318, index #4=w317, index #5=w316, index #6=w315) -> (element #1=w327:u16, element #3=w328:u16, element #4=w329:u16, element #5=w330:u16, element #6=w331:u16)  [unwired: 1 out]
              n161 = call "BRig_RT__Case_Exp__State_initTrial__LC.vi"("input_L_OnOff"=w327, "input_L_Block"=w311, "input_L_Count"=w328, "input_L_Prob"=w329, "input_L_Tdelay"=w330, "input_L_delayOpt"=w331, "input_T_state"=w326, "input_iSpout"=w311, "input_iTrial_relative"=w325, "input_L_T"=w312) -> ("output_LC_Event"=w322:bool, "output_LC_Laser"=w324:bool, "output_L_Tstart"=w323:u16, "output_L_Tend"=w321:u16)  [unwired: 6 in]
            }
            frame 3 {
              # "laser1 and laser2 are active"
              n162 = Index Array(array=w368, index #1=w347, index #2=w346, index #3=w345, index #4=w344, index #5=w343, index #6=w342, index #7=w341, index #8=w340, index #9=w339, index #10=w338, index #11=w337, index #12=w336) -> (element #1=w367:u16, element #3=w366:u16, element #4=w365:u16, element #5=w364:u16, element #6=w363:u16, element #7=w358:u16, element #9=w359:u16, element #10=w360:u16, element #11=w361:u16, element #12=w362:u16)  [unwired: 2 out]
              n163 = call "BRig_RT__Case_Exp__State_initTrial__LC.vi"("input_L_OnOff"=w367, "input_L_Block"=w333, "input_L_Count"=w366, "input_L_Prob"=w365, "input_L_Tdelay"=w364, "input_L_delayOpt"=w363, "input_T_state"=w357, "input_iSpout"=w333, "input_iTrial_relative"=w356, "input_L_T"=w335) -> ("output_LC_Event"=w355:bool, "output_LC_Laser"=w354:bool, "output_L_Tstart"=w353:u16, "output_L_Tend"=w352:u16)  [unwired: 6 in]
              n164 = call "BRig_RT__Case_Exp__State_initTrial__LC.vi"("input_L_OnOff"=w358, "input_L_Block"=w333, "input_L_Count"=w359, "input_L_Prob"=w360, "input_L_Tdelay"=w361, "input_L_delayOpt"=w362, "input_T_state"=w357, "input_iSpout"=w333, "input_iTrial_relative"=w356, "input_L_T"=w334) -> ("output_LC_Event"=w349:bool, "output_LC_Laser"=w351:bool, "output_L_Tstart"=w350:u16, "output_L_Tend"=w348:u16)  [unwired: 6 in]
            }
          }
          n165 = call "BRig_dataCurrent_L_Cue_T_start_l1.vi"() -> ("outputL_Cue_T_start_l1"=w48:i32)  [unwired: 11 in]
          n166 = call "BRig_dataCurrent_L_Cue_T_end_l1.vi"() -> ("output_L_Cue_T_end_l1"=w45:i32)  [unwired: 11 in]
          n167 = call "BRig_dataCurrent_L_Cue_T_start_l2.vi"() -> ("output_L_Cue_T_start_l2"=w46:i32)  [unwired: 11 in]
          n168 = call "BRig_dataCurrent_L_Cue_T_end_l2.vi"() -> ("output_L_Cue_T_end_l2"=w47:i32)  [unwired: 11 in]
          n169 = call "BRig_dataCurrent_L_Cue2_T_start_l1.vi"() -> ("outputL_Cue2_T_start_l1"=w44:i32)  [unwired: 11 in]
          n170 = call "BRig_dataCurrent_L_Cue2_T_end_l1.vi"() -> ("output_L_Cue2_T_end_l1"=w41:i32)  [unwired: 11 in]
          n171 = call "BRig_dataCurrent_L_Cue2_T_start_l2.vi"() -> ("output_L_Cue2_T_start_l2"=w42:i32)  [unwired: 11 in]
          n172 = call "BRig_dataCurrent_L_Cue2_T_end_l2.vi"() -> ("output_L_Cue2_T_end_l2"=w43:i32)  [unwired: 11 in]
          n173 = Replace Array Subset(array=w125, new element #1=w123, index #1=w48, new element #2=w122, index #2=w45, new element #3=w121, index #3=w46, new element #4=w120, index #4=w47, new element #5=w89, index #5=w44, new element #6=w88, index #6=w41, new element #7=w87, index #7=w42, new element #8=w86, index #8=w43) -> (w124:u16[])
          n174 = call "BRig_dataTrial_L_Cue_event_I_l1.vi"() -> ("output_L_Cue_event_I_l1"=w32:i32)  [unwired: 11 in]
          n175 = call "BRig_dataTrial_L_Cue_trig_I_l1.vi"() -> ("output_L_Cue_trig_I_l1"=w31:i32)  [unwired: 11 in]
          n176 = call "BRig_dataTrial_L_Cue_event_I_l2.vi"() -> ("output_L_Cue_event_I_l2"=w30:i32)  [unwired: 11 in]
          n177 = call "BRig_dataTrial_L_Cue_trig_I_l2.vi"() -> ("output_L_Cue_trig_I_l2"=w29:i32)  [unwired: 11 in]
          n178 = call "BRig_dataTrial_L_Cue2_event_I_l1.vi"() -> ("output_L_Cue2_event_I_l1"=w28:i32)  [unwired: 11 in]
          n179 = call "BRig_dataTrial_L_Cue2_trig_I_l1.vi"() -> ("output_L_Cue2_trig_I_l1"=w27:i32)  [unwired: 11 in]
          n180 = call "BRig_dataTrial_L_Cue2_event_I_l2.vi"() -> ("output_L_Cue2_event_I_l2"=w26:i32)  [unwired: 11 in]
          n181 = call "BRig_dataTrial_L_Cue2_trig_I_l2.vi"() -> ("output_L_Cue2_trig_I_l2"=w25:i32)  [unwired: 11 in]
          n182 = call "BRig_arrTrig_L_Cue_event_l1.vi"() -> ("output_L_Cue_event_l1"=w39:i32)  [unwired: 11 in]
          n183 = call "BRig_arrTrig_L_Cue_laser_l1.vi"() -> ("output_L_Cue_laser_l1"=w38:i32)  [unwired: 11 in]
          n184 = call "BRig_arrTrig_L_Cue_event_l2.vi"() -> ("output_L_Cue_event_l2"=w37:i32)  [unwired: 11 in]
          n185 = call "BRig_arrTrig_L_Cue_laser_l2.vi"() -> ("output_L_Cue_laser_l2"=w36:i32)  [unwired: 11 in]
          n186 = call "BRig_arrTrig_L_Cue2_event_l1.vi"() -> ("output_L_Cue2_event_l1"=w35:i32)  [unwired: 11 in]
          n187 = call "BRig_arrTrig_L_Cue2_laser_l1.vi"() -> ("output_L_Cue2_laser_l1"=w34:i32)  [unwired: 11 in]
          n188 = call "BRig_arrTrig_L_Cue2_event_l2.vi"() -> ("output_L_Cue2_event_l2"=w33:i32)  [unwired: 11 in]
          n189 = call "BRig_arrTrig_L_Cue2_laser_l2.vi"() -> ("output_L_Cue2_laser_l2"=w40:i32)  [unwired: 11 in]
          n190 = Boolean To (0,1)(Boolean=w134) -> (0, 1=w138:i16)
          n191 = Boolean To (0,1)(Boolean=w131) -> (0, 1=w137:i16)
          n192 = Boolean To (0,1)(Boolean=w129) -> (0, 1=w135:i16)
          n193 = Boolean To (0,1)(Boolean=w127) -> (0, 1=w136:i16)
          n194 = Boolean To (0,1)(Boolean=w93) -> (0, 1=w104:i16)
          n195 = Boolean To (0,1)(Boolean=w92) -> (0, 1=w103:i16)
          n196 = Boolean To (0,1)(Boolean=w91) -> (0, 1=w101:i16)
          n197 = Boolean To (0,1)(Boolean=w90) -> (0, 1=w102:i16)
          n198 = Replace Array Subset(array=w140, new element #1=w134, index #1=w39, new element #2=w131, index #2=w38, new element #3=w129, index #3=w37, new element #4=w127, index #4=w36, new element #5=w93, index #5=w35, new element #6=w92, index #6=w34, new element #7=w91, index #7=w33, new element #8=w90, index #8=w40) -> (w139:bool[])
          n199 = To Unsigned Word Integer(number=w138) -> (unsigned 16bit integer=w133:u16)
          n200 = To Unsigned Word Integer(number=w137) -> (unsigned 16bit integer=w132:u16)
          n201 = To Unsigned Word Integer(number=w135) -> (unsigned 16bit integer=w130:u16)
          n202 = To Unsigned Word Integer(number=w136) -> (unsigned 16bit integer=w128:u16)
          n203 = To Unsigned Word Integer(number=w104) -> (unsigned 16bit integer=w99:u16)
          n204 = To Unsigned Word Integer(number=w103) -> (unsigned 16bit integer=w98:u16)
          n205 = To Unsigned Word Integer(number=w101) -> (unsigned 16bit integer=w97:u16)
          n206 = To Unsigned Word Integer(number=w102) -> (unsigned 16bit integer=w96:u16)
          n207 = Replace Array Subset(array=w85, new element #1=w133, index (row) #1=w100, index (col) #1=w32, new element #2=w132, index (row) #2=w100, index (col) #2=w31, new element #3=w130, index (row) #3=w100, index (col) #3=w30, new element #4=w128, index (row) #4=w100, index (col) #4=w29, new element #5=w99, index (row) #5=w100, index (col) #5=w28, new element #6=w98, index (row) #6=w100, index (col) #6=w27, new element #7=w97, index (row) #7=w100, index (col) #7=w26, new element #8=w96, index (row) #8=w100, index (col) #8=w25) -> (w126:u16[][])
        }
        frame False {
          w512 = u16 1
          w538 = u16 0
          w539 = u16 2 ("input_sState_start")
          w561 = 0
          # "dataLC_Cue2_ [ ]\nnot used anymore"
          # "Need to force block condition to pass\nby setting iSpout = Block\nwhere Block is Block parameter\nfor both l1 and l2, and Reward and Wrong"
          # "Record laser timing"
          # "Calculate laser timing"
          # "Total Time (Cue2)"
          # "Total Time (Cue)"
          # "iTrial\nrelative"
          # "Total Time (Laser 2)"
          # "Total Time (Laser 1)"
          # "laser timing case (Cue2)"
          # "Determine case for\ncalculating laser timing"
          # "2) Get relative iTrial"
          # "1) If Trial Start State = PostReward,\nThen check LC_Cue_nReward"
          # "laser2 active (Cue2)?"
          # "laser1 active (Cue2)?"
          # "laser2 active (Cue)?"
          # "laser1 active (Cue)?"
          # "1) If Trial Start State = PostReward,\nThen check LC_Cue_nReward\n\n2) Get relative iTrial"
          # "Gather variables"
          # "Last trial's\niReward\n(0 = not reward)"
          # "idx dataTrial"
          # "Total Time (Cue2)"
          # "Total Time (Cue)"
          # "Have Cue2?"
          # "Total Time (Laser 2)"
          # "Total Time (Laser 1)"
          # "Calculate settings for Cue2"
          # "Calculate settings for Cue"
          # "Set laser settings for Cue and Cue2"
          # "iTrial\nrelative"
          # "laser timing case (Cue)"
          # "Trial start state\n0 (unknown)\n1 (first)\n2 (PreReward)\n3 (PostReward)"
          # "laser2 active?"
          # "laser1 active?"
          n208 = call "BRig_dataCurrent_LaserSwitch_l1.vi"() -> ("output_LaserSwitch_l1"=w597:i32)  [unwired: 11 in]
          n209 = call "BRig_dataCurrent_LaserSwitch_l2.vi"() -> ("output_LaserSwitch_l2"=w596:i32)  [unwired: 11 in]
          n210 = call "BRig_dataCurrent_T_Cue.vi"() -> ("output_T_Cue"=w537:i32)  [unwired: 11 in]
          n211 = call "BRig_dataCurrent_T_Cue2.vi"() -> ("output_T_Cue2"=w536:i32)  [unwired: 11 in]
          n212 = call "BRig_dataExp_L_Ttotal_l1.vi"() -> ("output_L_Ttotal_l1"=w567:i32)  [unwired: 11 in]
          n213 = call "BRig_dataExp_L_Ttotal_l2.vi"() -> ("output_L_Ttotal_l2"=w568:i32)  [unwired: 11 in]
          n214 = Index Array(array=w574, index #1=w597, index #2=w596, index #3=w537, index #4=w536) -> (element #1=w595:u16, element #2=w594:u16, element #3=w534:u16, element #4=w535:u16)
          n215 = Index Array(array=w566, index #1=w567, index #2=w568) -> (element #1=w556:u16, element #2=w555:u16)
          n216 = Not Equal To 0?(x=w595) -> (x != 0?=w532:bool)
          n217 = Not Equal To 0?(x=w594) -> (x != 0?=w531:bool)
          n218 = case shown="3" w512 {
            tunnel: u16 0 -> [_ _ w684]
            tunnel: w529 -> [_ _ w685]
            tunnel: w531 -> [_ w674 w677]
            tunnel: w532 -> [_ w675 w678]
            tunnel: w533 -> [_ w673 w676]
            tunnel: [w670 w675 w683] -> w528
            tunnel: [w670 w674 w682] -> w527
            tunnel: [w670 w672 w681] -> w526
            tunnel: [w670 w671 w680] -> w525
            frame 0 {
              w670 = FALSE
            }
            frame 1, Default {
              n219 = And(x=w673, y=w675) -> (x .and. y?=w672:bool)
              n220 = And(x=w674, y=w673) -> (x .and. y?=w671:bool)
            }
            frame 3 {
              w690 = i16 0 ("f")
              n221 = Boolean To (0,1)(Boolean=w678) -> (0, 1=w688:i16)
              n222 = Select(t=i16 2, s=w677, f=w690) -> (s? t:f=w689:i16)
              n223 = Select(t=i16 4, s=w676, f=w690) -> (s? t:f=w687:i16)
              n224 = Compound Arithmetic op=ADD(w688, w689, w687) -> (w686:i16)
              n225 = case shown="7" w686 {
                tunnel: w685 -> [_ w699 w710 w724 _ w749 w770 w797]
                tunnel: w684 -> [_ w698 w709 w723 _ w745 w766 w786]
                tunnel: [w693 w697 w707 w722 w735 w744 w763 w785] -> w683
                tunnel: [w693 w696 w708 w721 w735 w742 w765 w784] -> w682
                tunnel: [w693 w696 w707 w720 w735 w743 w763 w783] -> w681
                tunnel: [w693 w696 w707 w720 w735 w742 w764 w782] -> w680
                tunnel: FALSE -> [w693 w696 w707 w720 w735 w742 w763 _]
                frame 0, Default {
                }
                frame 1 {
                  n226 = call "BRig_dataLC_Cue_PostR_nRew1_l1.vi"() -> ("output_Cue_PostR_nRew1_l1"=w694:i32)  [unwired: 11 in]
                  n227 = call "BRig_dataLC_Cue_PostR_nRew2_l1.vi"() -> ("output_Cue_PostR_nRew2_l1"=w695:i32)  [unwired: 11 in]
                  n228 = Index Array(array=w699, index #1=w694, index #2=w695) -> (element #1=w701:u16, element #2=w700:u16)
                  n229 = Equal To 0?(x=w701) -> (x = 0?=w702:bool)
                  n230 = Equal?(x=w701, y=w698) -> (x = y?=w703:bool)
                  n231 = Equal?(x=w700, y=w698) -> (x = y?=w704:bool)
                  n232 = Compound Arithmetic op=OR(w702, w703, w704) -> (w697:bool)
                }
                frame 2 {
                  n233 = call "BRig_dataLC_Cue_PostR_nRew1_l2.vi"() -> ("output_Cue_PostR_nRew1_l2"=w705:i32)  [unwired: 11 in]
                  n234 = call "BRig_dataLC_Cue_PostR_nRew2_l2.vi"() -> ("output_Cue_PostR_nRew2_l2"=w706:i32)  [unwired: 11 in]
                  n235 = Index Array(array=w710, index #1=w705, index #2=w706) -> (element #1=w711:u16, element #2=w712:u16)
                  n236 = Equal To 0?(x=w711) -> (x = 0?=w714:bool)
                  n237 = Equal?(x=w711, y=w709) -> (x = y?=w713:bool)
                  n238 = Equal?(x=w712, y=w709) -> (x = y?=w715:bool)
                  n239 = Compound Arithmetic op=OR(w714, w713, w715) -> (w708:bool)
                }
                frame 3 {
                  n240 = call "BRig_dataLC_Cue_PostR_nRew1_l1.vi"() -> ("output_Cue_PostR_nRew1_l1"=w716:i32)  [unwired: 11 in]
                  n241 = call "BRig_dataLC_Cue_PostR_nRew2_l1.vi"() -> ("output_Cue_PostR_nRew2_l1"=w717:i32)  [unwired: 11 in]
                  n242 = call "BRig_dataLC_Cue_PostR_nRew1_l2.vi"() -> ("output_Cue_PostR_nRew1_l2"=w718:i32)  [unwired: 11 in]
                  n243 = call "BRig_dataLC_Cue_PostR_nRew2_l2.vi"() -> ("output_Cue_PostR_nRew2_l2"=w719:i32)  [unwired: 11 in]
                  n244 = Index Array(array=w724, index #1=w716, index #2=w717, index #3=w718, index #4=w719) -> (element #1=w728:u16, element #2=w727:u16, element #3=w725:u16, element #4=w726:u16)
                  n245 = Equal To 0?(x=w728) -> (x = 0?=w729:bool)
                  n246 = Equal?(x=w728, y=w723) -> (x = y?=w730:bool)
                  n247 = Equal?(x=w727, y=w723) -> (x = y?=w731:bool)
                  n248 = Equal To 0?(x=w725) -> (x = 0?=w733:bool)
                  n249 = Equal?(x=w725, y=w723) -> (x = y?=w732:bool)
                  n250 = Equal?(x=w726, y=w723) -> (x = y?=w734:bool)
                  n251 = Compound Arithmetic op=OR(w729, w730, w731) -> (w722:bool)
                  n252 = Compound Arithmetic op=OR(w733, w732, w734) -> (w721:bool)
                }
                frame 4 {
                }
                frame 5 {
                  n253 = call "BRig_dataLC_Cue_PostR_nRew1_l1.vi"() -> ("output_Cue_PostR_nRew1_l1"=w738:i32)  [unwired: 11 in]
                  n254 = call "BRig_dataLC_Cue_PostR_nRew2_l1.vi"() -> ("output_Cue_PostR_nRew2_l1"=w739:i32)  [unwired: 11 in]
                  n255 = call "BRig_dataLC_Cue2_PostR_nRew1_l1.vi"() -> ("output_Cue2_PostR_nRew1_l1"=w736:i32)  [unwired: 11 in]
                  n256 = call "BRig_dataLC_Cue2_PostR_nRew2_l1.vi"() -> ("output_Cue2_PostR_nRew2_l1"=w737:i32)  [unwired: 11 in]
                  n257 = Index Array(array=w749, index #1=w738, index #2=w739, index #3=w736, index #4=w737) -> (element #1=w751:u16, element #2=w750:u16, element #3=w741:u16, element #4=w740:u16)
                  n258 = Equal To 0?(x=w751) -> (x = 0?=w752:bool)
                  n259 = Equal?(x=w751, y=w745) -> (x = y?=w753:bool)
                  n260 = Equal?(x=w750, y=w745) -> (x = y?=w754:bool)
                  n261 = Equal To 0?(x=w741) -> (x = 0?=w748:bool)
                  n262 = Equal?(x=w741, y=w745) -> (x = y?=w747:bool)
                  n263 = Equal?(x=w740, y=w745) -> (x = y?=w746:bool)
                  n264 = Compound Arithmetic op=OR(w752, w753, w754) -> (w744:bool)
                  n265 = Compound Arithmetic op=OR(w748, w747, w746) -> (w743:bool)
                }
                frame 6 {
                  n266 = call "BRig_dataLC_Cue_PostR_nRew1_l2.vi"() -> ("output_Cue_PostR_nRew1_l2"=w758:i32)  [unwired: 11 in]
                  n267 = call "BRig_dataLC_Cue_PostR_nRew2_l2.vi"() -> ("output_Cue_PostR_nRew2_l2"=w757:i32)  [unwired: 11 in]
                  n268 = call "BRig_dataLC_Cue2_PostR_nRew1_l2.vi"() -> ("output_Cue2_PostR_nRew1_l2"=w756:i32)  [unwired: 11 in]
                  n269 = call "BRig_dataLC_Cue2_PostR_nRew2_l2.vi"() -> ("output_Cue2_PostR_nRew2_l2"=w755:i32)  [unwired: 11 in]
                  n270 = Index Array(array=w770, index #1=w758, index #2=w757, index #3=w756, index #4=w755) -> (element #1=w762:u16, element #2=w761:u16, element #3=w760:u16, element #4=w759:u16)
                  n271 = Equal To 0?(x=w762) -> (x = 0?=w772:bool)
                  n272 = Equal?(x=w762, y=w766) -> (x = y?=w771:bool)
                  n273 = Equal?(x=w761, y=w766) -> (x = y?=w773:bool)
                  n274 = Equal To 0?(x=w760) -> (x = 0?=w768:bool)
                  n275 = Equal?(x=w760, y=w766) -> (x = y?=w769:bool)
                  n276 = Equal?(x=w759, y=w766) -> (x = y?=w767:bool)
                  n277 = Compound Arithmetic op=OR(w772, w771, w773) -> (w765:bool)
                  n278 = Compound Arithmetic op=OR(w768, w769, w767) -> (w764:bool)
                }
                frame 7 {
                  n279 = call "BRig_dataLC_Cue_PostR_nRew1_l1.vi"() -> ("output_Cue_PostR_nRew1_l1"=w778:i32)  [unwired: 11 in]
                  n280 = call "BRig_dataLC_Cue_PostR_nRew2_l1.vi"() -> ("output_Cue_PostR_nRew2_l1"=w779:i32)  [unwired: 11 in]
                  n281 = call "BRig_dataLC_Cue_PostR_nRew1_l2.vi"() -> ("output_Cue_PostR_nRew1_l2"=w780:i32)  [unwired: 11 in]
                  n282 = call "BRig_dataLC_Cue_PostR_nRew2_l2.vi"() -> ("output_Cue_PostR_nRew2_l2"=w781:i32)  [unwired: 11 in]
                  n283 = call "BRig_dataLC_Cue2_PostR_nRew1_l1.vi"() -> ("output_Cue2_PostR_nRew1_l1"=w777:i32)  [unwired: 11 in]
                  n284 = call "BRig_dataLC_Cue2_PostR_nRew2_l1.vi"() -> ("output_Cue2_PostR_nRew2_l1"=w776:i32)  [unwired: 11 in]
                  n285 = call "BRig_dataLC_Cue2_PostR_nRew1_l2.vi"() -> ("output_Cue2_PostR_nRew1_l2"=w775:i32)  [unwired: 11 in]
                  n286 = call "BRig_dataLC_Cue2_PostR_nRew2_l2.vi"() -> ("output_Cue2_PostR_nRew2_l2"=w774:i32)  [unwired: 11 in]
                  n287 = Index Array(array=w797, index #1=w778, index #2=w779, index #3=w780, index #4=w781, index #5=w777, index #6=w776, index #7=w775, index #8=w774) -> (element #1=w801:u16, element #2=w800:u16, element #3=w798:u16, element #4=w799:u16, element #5=w790:u16, element #6=w789:u16, element #7=w787:u16, element #8=w788:u16)
                  n288 = Equal To 0?(x=w801) -> (x = 0?=w802:bool)
                  n289 = Equal?(x=w801, y=w786) -> (x = y?=w803:bool)
                  n290 = Equal?(x=w800, y=w786) -> (x = y?=w804:bool)
                  n291 = Equal To 0?(x=w798) -> (x = 0?=w806:bool)
                  n292 = Equal?(x=w798, y=w786) -> (x = y?=w805:bool)
                  n293 = Equal?(x=w799, y=w786) -> (x = y?=w807:bool)
                  n294 = Equal To 0?(x=w790) -> (x = 0?=w796:bool)
                  n295 = Equal?(x=w790, y=w786) -> (x = y?=w795:bool)
                  n296 = Equal?(x=w789, y=w786) -> (x = y?=w794:bool)
                  n297 = Equal To 0?(x=w787) -> (x = 0?=w792:bool)
                  n298 = Equal?(x=w787, y=w786) -> (x = y?=w793:bool)
                  n299 = Equal?(x=w788, y=w786) -> (x = y?=w791:bool)
                  n300 = Compound Arithmetic op=OR(w802, w803, w804) -> (w785:bool)
                  n301 = Compound Arithmetic op=OR(w806, w805, w807) -> (w784:bool)
                  n302 = Compound Arithmetic op=OR(w796, w795, w794) -> (w783:bool)
                  n303 = Compound Arithmetic op=OR(w792, w793, w791) -> (w782:bool)
                }
              }
            }
          }
          n304 = case shown="1, Default" w512 {
            tunnel: [w634 w657 w668] -> w524
            tunnel: [w635 w646 w667] -> w523
            tunnel: [w636 w647 w666] -> w522
            tunnel: [w637 w648 w665] -> w521
            tunnel: [w638 w649 w664] -> w520
            tunnel: [w639 w650 w663] -> w519
            tunnel: [w640 w656 w662] -> w518
            tunnel: [w641 w651 w661] -> w517
            tunnel: [w642 w652 w660] -> w516
            tunnel: [w643 w653 w659] -> w515
            tunnel: [w644 w654 w658] -> w514
            tunnel: [w645 w655 w669] -> w513
            frame 1, Default {
              n305 = call "BRig_dataLC_Cue_First_OnOff_l1.vi"() -> ("output_Cue_First_OnOff"=w634:i32)  [unwired: 11 in]
              n306 = call "BRig_dataLC_Cue_First_Block_l1.vi"() -> ("output_Cue_First_Block"=w635:i32)  [unwired: 11 in]
              n307 = call "BRig_dataLC_Cue_First_Count_l1.vi"() -> ("output_Cue_First_Count"=w636:i32)  [unwired: 11 in]
              n308 = call "BRig_dataLC_Cue_First_Prob_l1.vi"() -> ("output_Cue_First_Prob"=w637:i32)  [unwired: 11 in]
              n309 = call "BRig_dataLC_Cue_First_Delay_l1.vi"() -> ("output_Cue_First_Delay"=w638:i32)  [unwired: 11 in]
              n310 = call "BRig_dataLC_Cue_First_DelayOpt_l1.vi"() -> ("output_Cue_First_DelayOpt"=w639:i32)  [unwired: 11 in]
              n311 = call "BRig_dataLC_Cue_First_OnOff_l2.vi"() -> ("output_Cue_First_OnOff_l2"=w640:i32)  [unwired: 11 in]
              n312 = call "BRig_dataLC_Cue_First_Block_l2.vi"() -> ("output_Cue_First_Block_l2"=w641:i32)  [unwired: 11 in]
              n313 = call "BRig_dataLC_Cue_First_Count_l2.vi"() -> ("output_Cue_First_Count_l2"=w642:i32)  [unwired: 11 in]
              n314 = call "BRig_dataLC_Cue_First_Prob_l2.vi"() -> ("output_Cue_First_Prob_l2"=w643:i32)  [unwired: 11 in]
              n315 = call "BRig_dataLC_Cue_First_Delay_l2.vi"() -> ("output_Cue_First_Delay_l2"=w644:i32)  [unwired: 11 in]
              n316 = call "BRig_dataLC_Cue_First_DelayOpt_l2.vi"() -> ("output_Cue_First_DelayOpt_l2"=w645:i32)  [unwired: 11 in]
            }
            frame 2 {
              n317 = call "BRig_dataLC_Cue_PreR_OnOff_l1.vi"() -> ("output_Cue_PreR_OnOff"=w657:i32)  [unwired: 11 in]
              n318 = call "BRig_dataLC_Cue_PreR_Block_l1.vi"() -> ("output_Cue_PreR_Block"=w646:i32)  [unwired: 11 in]
              n319 = call "BRig_dataLC_Cue_PreR_Count_l1.vi"() -> ("output_Cue_PreR_Count"=w647:i32)  [unwired: 11 in]
              n320 = call "BRig_dataLC_Cue_PreR_Prob_l1.vi"() -> ("output_Cue_PreR_Prob"=w648:i32)  [unwired: 11 in]
              n321 = call "BRig_dataLC_Cue_PreR_Delay_l1.vi"() -> ("output_Cue_PreR_Delay"=w649:i32)  [unwired: 11 in]
              n322 = call "BRig_dataLC_Cue_PreR_DelayOpt_l1.vi"() -> ("output_Cue_PreR_DelayOpt"=w650:i32)  [unwired: 11 in]
              n323 = call "BRig_dataLC_Cue_PreR_OnOff_l2.vi"() -> ("output_Cue_PreR_OnOff_l2"=w656:i32)  [unwired: 11 in]
              n324 = call "BRig_dataLC_Cue_PreR_Block_l2.vi"() -> ("output_Cue_PreR_Block_l2"=w651:i32)  [unwired: 11 in]
              n325 = call "BRig_dataLC_Cue_PreR_Count_l2.vi"() -> ("output_Cue_PreR_Count_l2"=w652:i32)  [unwired: 11 in]
              n326 = call "BRig_dataLC_Cue_PreR_Prob_l2.vi"() -> ("output_Cue_PreR_Prob_l2"=w653:i32)  [unwired: 11 in]
              n327 = call "BRig_dataLC_Cue_PreR_Delay_l2.vi"() -> ("output_Cue_PreR_Delay_l2"=w654:i32)  [unwired: 11 in]
              n328 = call "BRig_dataLC_Cue_PreR_DelayOpt_l2.vi"() -> ("output_Cue_PreR_DelayOpt_l2"=w655:i32)  [unwired: 11 in]
            }
            frame 3 {
              n329 = call "BRig_dataLC_Cue_PostR_OnOff_l1.vi"() -> ("output_Cue_PostR_OnOff"=w668:i32)  [unwired: 11 in]
              n330 = call "BRig_dataLC_Cue_PostR_Block_l1.vi"() -> ("output_Cue_PostR_Block"=w667:i32)  [unwired: 11 in]
              n331 = call "BRig_dataLC_Cue_PostR_Count_l1.vi"() -> ("output_Cue_PostR_Count"=w666:i32)  [unwired: 11 in]
              n332 = call "BRig_dataLC_Cue_PostR_Prob_l1.vi"() -> ("output_Cue_PostR_Prob"=w665:i32)  [unwired: 11 in]
              n333 = call "BRig_dataLC_Cue_PostR_Delay_l1.vi"() -> ("output_Cue_PostR_Delay"=w664:i32)  [unwired: 11 in]
              n334 = call "BRig_dataLC_Cue_PostR_DelayOpt_l1.vi"() -> ("output_Cue_PostR_DelayOpt"=w663:i32)  [unwired: 11 in]
              n335 = call "BRig_dataLC_Cue_PostR_OnOff_l2.vi"() -> ("output_Cue_PostR_OnOff_l2"=w662:i32)  [unwired: 11 in]
              n336 = call "BRig_dataLC_Cue_PostR_Block_l2.vi"() -> ("output_Cue_PostR_Block_l2"=w661:i32)  [unwired: 11 in]
              n337 = call "BRig_dataLC_Cue_PostR_Count_l2.vi"() -> ("output_Cue_PostR_Count_l2"=w660:i32)  [unwired: 11 in]
              n338 = call "BRig_dataLC_Cue_PostR_Prob_l2.vi"() -> ("output_Cue_PostR_Prob_l2"=w659:i32)  [unwired: 11 in]
              n339 = call "BRig_dataLC_Cue_PostR_Delay_l2.vi"() -> ("output_Cue_PostR_Delay_l2"=w658:i32)  [unwired: 11 in]
              n340 = call "BRig_dataLC_Cue_PostR_DelayOpt_l2.vi"() -> ("output_Cue_PostR_DelayOpt_l2"=w669:i32)  [unwired: 11 in]
            }
          }
          n341 = case shown="3" w512 {
            tunnel: [w609 w621 w633] -> w511
            tunnel: [w608 w620 w632] -> w510
            tunnel: [w607 w619 w631] -> w509
            tunnel: [w606 w618 w630] -> w508
            tunnel: [w605 w617 w629] -> w507
            tunnel: [w604 w616 w628] -> w506
            tunnel: [w603 w615 w627] -> w505
            tunnel: [w602 w614 w626] -> w504
            tunnel: [w601 w613 w625] -> w503
            tunnel: [w600 w612 w624] -> w502
            tunnel: [w599 w611 w623] -> w501
            tunnel: [w598 w610 w622] -> w500
            frame 1, Default {
              n342 = call "BRig_dataLC_Cue2_First_OnOff_l1.vi"() -> ("output_Cue2_First_OnOff"=w609:i32)  [unwired: 11 in]
              n343 = call "BRig_dataLC_Cue2_First_Block_l1.vi"() -> ("output_Cue2_First_Block"=w608:i32)  [unwired: 11 in]
              n344 = call "BRig_dataLC_Cue2_First_Count_l1.vi"() -> ("output_Cue2_First_Count"=w607:i32)  [unwired: 11 in]
              n345 = call "BRig_dataLC_Cue2_First_Prob_l1.vi"() -> ("output_Cue2_First_Prob"=w606:i32)  [unwired: 11 in]
              n346 = call "BRig_dataLC_Cue2_First_Delay_l1.vi"() -> ("output_Cue2_First_Delay"=w605:i32)  [unwired: 11 in]
              n347 = call "BRig_dataLC_Cue2_First_DelayOpt_l1.vi"() -> ("output_Cue2_First_DelayOpt"=w604:i32)  [unwired: 11 in]
              n348 = call "BRig_dataLC_Cue2_First_OnOff_l2.vi"() -> ("output_Cue2_First_OnOff_l2"=w603:i32)  [unwired: 11 in]
              n349 = call "BRig_dataLC_Cue2_First_Block_l2.vi"() -> ("output_Cue2_First_Block_l2"=w602:i32)  [unwired: 11 in]
              n350 = call "BRig_dataLC_Cue2_First_Count_l2.vi"() -> ("output_Cue2_First_Count_l2"=w601:i32)  [unwired: 11 in]
              n351 = call "BRig_dataLC_Cue2_First_Prob_l2.vi"() -> ("output_Cue2_First_Prob_l2"=w600:i32)  [unwired: 11 in]
              n352 = call "BRig_dataLC_Cue2_First_Delay_l2.vi"() -> ("output_Cue2_First_Delay_l2"=w599:i32)  [unwired: 11 in]
              n353 = call "BRig_dataLC_Cue2_First_DelayOpt_l2.vi"() -> ("output_Cue2_First_DelayOpt_l2"=w598:i32)  [unwired: 11 in]
            }
            frame 2 {
              n354 = call "BRig_dataLC_Cue2_PreR_OnOff_l1.vi"() -> ("output_Cue2_PreR_OnOff"=w621:i32)  [unwired: 11 in]
              n355 = call "BRig_dataLC_Cue2_PreR_Block_l1.vi"() -> ("output_Cue2_PreR_Block"=w620:i32)  [unwired: 11 in]
              n356 = call "BRig_dataLC_Cue2_PreR_Count_l1.vi"() -> ("output_Cue2_PreR_Count"=w619:i32)  [unwired: 11 in]
              n357 = call "BRig_dataLC_Cue2_PreR_Prob_l1.vi"() -> ("output_Cue2_PreR_Prob"=w618:i32)  [unwired: 11 in]
              n358 = call "BRig_dataLC_Cue2_PreR_Delay_l1.vi"() -> ("output_Cue2_PreR_Delay"=w617:i32)  [unwired: 11 in]
              n359 = call "BRig_dataLC_Cue2_PreR_DelayOpt_l1.vi"() -> ("output_Cue2_PreR_DelayOpt"=w616:i32)  [unwired: 11 in]
              n360 = call "BRig_dataLC_Cue2_PreR_OnOff_l2.vi"() -> ("output_Cue2_PreR_OnOff_l2"=w615:i32)  [unwired: 11 in]
              n361 = call "BRig_dataLC_Cue2_PreR_Block_l2.vi"() -> ("output_Cue2_PreR_Block_l2"=w614:i32)  [unwired: 11 in]
              n362 = call "BRig_dataLC_Cue2_PreR_Count_l2.vi"() -> ("output_Cue2_PreR_Count_l2"=w613:i32)  [unwired: 11 in]
              n363 = call "BRig_dataLC_Cue2_PreR_Prob_l2.vi"() -> ("output_Cue2_PreR_Prob_l2"=w612:i32)  [unwired: 11 in]
              n364 = call "BRig_dataLC_Cue2_PreR_Delay_l2.vi"() -> ("output_Cue2_PreR_Delay_l2"=w611:i32)  [unwired: 11 in]
              n365 = call "BRig_dataLC_Cue2_PreR_DelayOpt_l2.vi"() -> ("output_Cue2_PreR_DelayOpt_l2"=w610:i32)  [unwired: 11 in]
            }
            frame 3 {
              n366 = call "BRig_dataLC_Cue2_PostR_OnOff_l1.vi"() -> ("output_Cue2_PostR_OnOff"=w633:i32)  [unwired: 11 in]
              n367 = call "BRig_dataLC_Cue2_PostR_Block_l1.vi"() -> ("output_Cue2_PostR_Block"=w632:i32)  [unwired: 11 in]
              n368 = call "BRig_dataLC_Cue2_PostR_Count_l1.vi"() -> ("output_Cue2_PostR_Count"=w631:i32)  [unwired: 11 in]
              n369 = call "BRig_dataLC_Cue2_PostR_Prob_l1.vi"() -> ("output_Cue2_PostR_Prob"=w630:i32)  [unwired: 11 in]
              n370 = call "BRig_dataLC_Cue2_PostR_Delay_l1.vi"() -> ("output_Cue2_PostR_Delay"=w629:i32)  [unwired: 11 in]
              n371 = call "BRig_dataLC_Cue2_PostR_DelayOpt_l1.vi"() -> ("output_Cue2_PostR_DelayOpt"=w628:i32)  [unwired: 11 in]
              n372 = call "BRig_dataLC_Cue2_PostR_OnOff_l2.vi"() -> ("output_Cue2_PostR_OnOff_l2"=w627:i32)  [unwired: 11 in]
              n373 = call "BRig_dataLC_Cue2_PostR_Block_l2.vi"() -> ("output_Cue2_PostR_Block_l2"=w626:i32)  [unwired: 11 in]
              n374 = call "BRig_dataLC_Cue2_PostR_Count_l2.vi"() -> ("output_Cue2_PostR_Count_l2"=w625:i32)  [unwired: 11 in]
              n375 = call "BRig_dataLC_Cue2_PostR_Prob_l2.vi"() -> ("output_Cue2_PostR_Prob_l2"=w624:i32)  [unwired: 11 in]
              n376 = call "BRig_dataLC_Cue2_PostR_Delay_l2.vi"() -> ("output_Cue2_PostR_Delay_l2"=w623:i32)  [unwired: 11 in]
              n377 = call "BRig_dataLC_Cue2_PostR_DelayOpt_l2.vi"() -> ("output_Cue2_PostR_DelayOpt_l2"=w622:i32)  [unwired: 11 in]
            }
          }
          n378 = Boolean To (0,1)(Boolean=w528) -> (0, 1=w591:i16)
          n379 = Boolean To (0,1)(Boolean=w526) -> (0, 1=w544:i16)
          n380 = Select(t=i16 2, s=w527, f=i16 0) -> (s? t:f=w592:i16)
          n381 = Select(t=i16 2, s=w525, f=i16 0) -> (s? t:f=w543:i16)
          n382 = Add(x=w591, y=w592) -> (x+y=w541:i16)
          n383 = Add(x=w544, y=w543) -> (x+y=w540:i16)
          n384 = case shown="1" w541 {
            tunnel: w529 -> [_ w913 w935 w972]
            tunnel: w539 -> [_ w892 w914 w936]
            tunnel: w534 -> [_ w907 w929 w960]
            tunnel: w538 -> [_ w906 w928 w959]
            tunnel: [w890 w905 w917 w958] -> w583
            tunnel: [w890 w904 w917 w957] -> w580
            tunnel: [w891 w903 w916 w956] -> w572
            tunnel: [w891 w902 w916 w955] -> w571
            tunnel: [w890 w895 w927 w954] -> w576
            tunnel: [w891 w894 w926 w953] -> w570
            tunnel: [w890 w895 w925 w952] -> w578
            tunnel: [w891 w894 w924 w951] -> w569
            tunnel: w524 -> [_ w901 _ w950]
            tunnel: w523 -> [_ w900 _ w949]
            tunnel: w522 -> [_ w899 _ w948]
            tunnel: w521 -> [_ w898 _ w947]
            tunnel: w520 -> [_ w897 _ w946]
            tunnel: w519 -> [_ w896 _ w945]
            tunnel: w518 -> [_ _ w923 w944]
            tunnel: w517 -> [_ _ w922 w943]
            tunnel: w516 -> [_ _ w921 w942]
            tunnel: w515 -> [_ _ w920 w941]
            tunnel: w514 -> [_ _ w919 w940]
            tunnel: w513 -> [_ _ w918 w939]
            tunnel: w556 -> [_ w893 _ w938]
            tunnel: w555 -> [_ _ w915 w937]
            frame 0, Default {
              w891 = u16 0
              w890 = FALSE
              # "No active lasers"
            }
            frame 1 {
              w894 = u16 0
              w895 = FALSE
              # "laser1 is active"
              n385 = Index Array(array=w913, index #1=w901, index #2=w900, index #3=w899, index #4=w898, index #5=w897, index #6=w896) -> (element #1=w912:u16, element #3=w911:u16, element #4=w910:u16, element #5=w909:u16, element #6=w908:u16)  [unwired: 1 out]
              n386 = call "BRig_RT__Case_Exp__State_initTrial__LC.vi"("input_L_OnOff"=w912, "input_L_Block"=w892, "input_L_Count"=w911, "input_L_Prob"=w910, "input_L_Tdelay"=w909, "input_L_delayOpt"=w908, "input_T_state"=w907, "input_iSpout"=w892, "input_iTrial_relative"=w906, "input_L_T"=w893) -> ("output_LC_Event"=w905:bool, "output_LC_Laser"=w904:bool, "output_L_Tstart"=w903:u16, "output_L_Tend"=w902:u16)  [unwired: 6 in]
            }
            frame 2 {
              w916 = u16 0
              w917 = FALSE
              # "laser2 is active"
              n387 = Index Array(array=w935, index #1=w923, index #2=w922, index #3=w921, index #4=w920, index #5=w919, index #6=w918) -> (element #1=w930:u16, element #3=w931:u16, element #4=w932:u16, element #5=w933:u16, element #6=w934:u16)  [unwired: 1 out]
              n388 = call "BRig_RT__Case_Exp__State_initTrial__LC.vi"("input_L_OnOff"=w930, "input_L_Block"=w914, "input_L_Count"=w931, "input_L_Prob"=w932, "input_L_Tdelay"=w933, "input_L_delayOpt"=w934, "input_T_state"=w929, "input_iSpout"=w914, "input_iTrial_relative"=w928, "input_L_T"=w915) -> ("output_LC_Event"=w925:bool, "output_LC_Laser"=w927:bool, "output_L_Tstart"=w926:u16, "output_L_Tend"=w924:u16)  [unwired: 6 in]
            }
            frame 3 {
              # "laser1 and laser2 are active"
              n389 = Index Array(array=w972, index #1=w950, index #2=w949, index #3=w948, index #4=w947, index #5=w946, index #6=w945, index #7=w944, index #8=w943, index #9=w942, index #10=w941, index #11=w940, index #12=w939) -> (element #1=w971:u16, element #2=w970:u16, element #3=w969:u16, element #4=w968:u16, element #5=w967:u16, element #6=w966:u16, element #7=w961:u16, element #9=w962:u16, element #10=w963:u16, element #11=w964:u16, element #12=w965:u16)  [unwired: 1 out]
              n390 = call "BRig_RT__Case_Exp__State_initTrial__LC.vi"("input_L_OnOff"=w971, "input_L_Block"=w970, "input_L_Count"=w969, "input_L_Prob"=w968, "input_L_Tdelay"=w967, "input_L_delayOpt"=w966, "input_T_state"=w960, "input_iSpout"=w936, "input_iTrial_relative"=w959, "input_L_T"=w938) -> ("output_LC_Event"=w958:bool, "output_LC_Laser"=w957:bool, "output_L_Tstart"=w956:u16, "output_L_Tend"=w955:u16)  [unwired: 6 in]
              n391 = call "BRig_RT__Case_Exp__State_initTrial__LC.vi"("input_L_OnOff"=w961, "input_L_Block"=w936, "input_L_Count"=w962, "input_L_Prob"=w963, "input_L_Tdelay"=w964, "input_L_delayOpt"=w965, "input_T_state"=w960, "input_iSpout"=w936, "input_iTrial_relative"=w959, "input_L_T"=w937) -> ("output_LC_Event"=w952:bool, "output_LC_Laser"=w954:bool, "output_L_Tstart"=w953:u16, "output_L_Tend"=w951:u16)  [unwired: 6 in]
            }
          }
          n392 = case shown="1" w540 {
            tunnel: w529 -> [_ w831 w853 w889]
            tunnel: w539 -> [_ w810 w832 w854]
            tunnel: w535 -> [_ w825 w847 w878]
            tunnel: w538 -> [_ w824 w846 w877]
            tunnel: [w808 w823 w835 w876] -> w554
            tunnel: [w808 w822 w835 w875] -> w553
            tunnel: [w809 w821 w834 w874] -> w550
            tunnel: [w809 w820 w834 w873] -> w549
            tunnel: [w808 w813 w845 w872] -> w551
            tunnel: [w809 w812 w844 w871] -> w548
            tunnel: [w808 w813 w843 w870] -> w552
            tunnel: [w809 w812 w842 w869] -> w547
            tunnel: w511 -> [_ w819 _ w868]
            tunnel: w510 -> [_ w818 _ w867]
            tunnel: w509 -> [_ w817 _ w866]
            tunnel: w508 -> [_ w816 _ w865]
            tunnel: w507 -> [_ w815 _ w864]
            tunnel: w506 -> [_ w814 _ w863]
            tunnel: w505 -> [_ _ w841 w862]
            tunnel: w504 -> [_ _ w840 w861]
            tunnel: w503 -> [_ _ w839 w860]
            tunnel: w502 -> [_ _ w838 w859]
            tunnel: w501 -> [_ _ w837 w858]
            tunnel: w500 -> [_ _ w836 w857]
            tunnel: w556 -> [_ w811 _ w856]
            tunnel: w555 -> [_ _ w833 w855]
            frame 0, Default {
              w809 = u16 0
              w808 = FALSE
              # "No active lasers"
            }
            frame 1 {
              w812 = u16 0
              w813 = FALSE
              # "laser1 is active"
              n393 = Index Array(array=w831, index #1=w819, index #2=w818, index #3=w817, index #4=w816, index #5=w815, index #6=w814) -> (element #1=w830:u16, element #3=w829:u16, element #4=w828:u16, element #5=w827:u16, element #6=w826:u16)  [unwired: 1 out]
              n394 = call "BRig_RT__Case_Exp__State_initTrial__LC.vi"("input_L_OnOff"=w830, "input_L_Block"=w810, "input_L_Count"=w829, "input_L_Prob"=w828, "input_L_Tdelay"=w827, "input_L_delayOpt"=w826, "input_T_state"=w825, "input_iSpout"=w810, "input_iTrial_relative"=w824, "input_L_T"=w811) -> ("output_LC_Event"=w823:bool, "output_LC_Laser"=w822:bool, "output_L_Tstart"=w821:u16, "output_L_Tend"=w820:u16)  [unwired: 6 in]
            }
            frame 2 {
              w834 = u16 0
              w835 = FALSE
              # "laser2 is active"
              n395 = Index Array(array=w853, index #1=w841, index #2=w840, index #3=w839, index #4=w838, index #5=w837, index #6=w836) -> (element #1=w848:u16, element #3=w849:u16, element #4=w850:u16, element #5=w851:u16, element #6=w852:u16)  [unwired: 1 out]
              n396 = call "BRig_RT__Case_Exp__State_initTrial__LC.vi"("input_L_OnOff"=w848, "input_L_Block"=w832, "input_L_Count"=w849, "input_L_Prob"=w850, "input_L_Tdelay"=w851, "input_L_delayOpt"=w852, "input_T_state"=w847, "input_iSpout"=w832, "input_iTrial_relative"=w846, "input_L_T"=w833) -> ("output_LC_Event"=w843:bool, "output_LC_Laser"=w845:bool, "output_L_Tstart"=w844:u16, "output_L_Tend"=w842:u16)  [unwired: 6 in]
            }
            frame 3 {
              # "laser1 and laser2 are active"
              n397 = Index Array(array=w889, index #1=w868, index #2=w867, index #3=w866, index #4=w865, index #5=w864, index #6=w863, index #7=w862, index #8=w861, index #9=w860, index #10=w859, index #11=w858, index #12=w857) -> (element #1=w888:u16, element #3=w887:u16, element #4=w886:u16, element #5=w885:u16, element #6=w884:u16, element #7=w879:u16, element #9=w880:u16, element #10=w881:u16, element #11=w882:u16, element #12=w883:u16)  [unwired: 2 out]
              n398 = call "BRig_RT__Case_Exp__State_initTrial__LC.vi"("input_L_OnOff"=w888, "input_L_Block"=w854, "input_L_Count"=w887, "input_L_Prob"=w886, "input_L_Tdelay"=w885, "input_L_delayOpt"=w884, "input_T_state"=w878, "input_iSpout"=w854, "input_iTrial_relative"=w877, "input_L_T"=w856) -> ("output_LC_Event"=w876:bool, "output_LC_Laser"=w875:bool, "output_L_Tstart"=w874:u16, "output_L_Tend"=w873:u16)  [unwired: 6 in]
              n399 = call "BRig_RT__Case_Exp__State_initTrial__LC.vi"("input_L_OnOff"=w879, "input_L_Block"=w854, "input_L_Count"=w880, "input_L_Prob"=w881, "input_L_Tdelay"=w882, "input_L_delayOpt"=w883, "input_T_state"=w878, "input_iSpout"=w854, "input_iTrial_relative"=w877, "input_L_T"=w855) -> ("output_LC_Event"=w870:bool, "output_LC_Laser"=w872:bool, "output_L_Tstart"=w871:u16, "output_L_Tend"=w869:u16)  [unwired: 6 in]
            }
          }
          n400 = call "BRig_dataCurrent_L_Cue_T_start_l1.vi"() -> ("outputL_Cue_T_start_l1"=w499:i32)  [unwired: 11 in]
          n401 = call "BRig_dataCurrent_L_Cue_T_end_l1.vi"() -> ("output_L_Cue_T_end_l1"=w498:i32)  [unwired: 11 in]
          n402 = call "BRig_dataCurrent_L_Cue_T_start_l2.vi"() -> ("output_L_Cue_T_start_l2"=w497:i32)  [unwired: 11 in]
          n403 = call "BRig_dataCurrent_L_Cue_T_end_l2.vi"() -> ("output_L_Cue_T_end_l2"=w496:i32)  [unwired: 11 in]
          n404 = call "BRig_dataCurrent_L_Cue2_T_start_l1.vi"() -> ("outputL_Cue2_T_start_l1"=w487:i32)  [unwired: 11 in]
          n405 = call "BRig_dataCurrent_L_Cue2_T_end_l1.vi"() -> ("output_L_Cue2_T_end_l1"=w484:i32)  [unwired: 11 in]
          n406 = call "BRig_dataCurrent_L_Cue2_T_start_l2.vi"() -> ("output_L_Cue2_T_start_l2"=w485:i32)  [unwired: 11 in]
          n407 = call "BRig_dataCurrent_L_Cue2_T_end_l2.vi"() -> ("output_L_Cue2_T_end_l2"=w486:i32)  [unwired: 11 in]
          n408 = Replace Array Subset(array=w574, new element #1=w572, index #1=w499, new element #2=w571, index #2=w498, new element #3=w570, index #3=w497, new element #4=w569, index #4=w496, new element #5=w550, index #5=w487, new element #6=w549, index #6=w484, new element #7=w548, index #7=w485, new element #8=w547, index #8=w486) -> (w573:u16[])
          n409 = call "BRig_dataTrial_L_Cue_event_I_l1.vi"() -> ("output_L_Cue_event_I_l1"=w483:i32)  [unwired: 11 in]
          n410 = call "BRig_dataTrial_L_Cue_trig_I_l1.vi"() -> ("output_L_Cue_trig_I_l1"=w482:i32)  [unwired: 11 in]
          n411 = call "BRig_dataTrial_L_Cue_event_I_l2.vi"() -> ("output_L_Cue_event_I_l2"=w481:i32)  [unwired: 11 in]
          n412 = call "BRig_dataTrial_L_Cue_trig_I_l2.vi"() -> ("output_L_Cue_trig_I_l2"=w480:i32)  [unwired: 11 in]
          n413 = call "BRig_dataTrial_L_Cue2_event_I_l1.vi"() -> ("output_L_Cue2_event_I_l1"=w479:i32)  [unwired: 11 in]
          n414 = call "BRig_dataTrial_L_Cue2_trig_I_l1.vi"() -> ("output_L_Cue2_trig_I_l1"=w478:i32)  [unwired: 11 in]
          n415 = call "BRig_dataTrial_L_Cue2_event_I_l2.vi"() -> ("output_L_Cue2_event_I_l2"=w477:i32)  [unwired: 11 in]
          n416 = call "BRig_dataTrial_L_Cue2_trig_I_l2.vi"() -> ("output_L_Cue2_trig_I_l2"=w476:i32)  [unwired: 11 in]
          n417 = call "BRig_arrTrig_L_Cue_event_l1.vi"() -> ("output_L_Cue_event_l1"=w494:i32)  [unwired: 11 in]
          n418 = call "BRig_arrTrig_L_Cue_laser_l1.vi"() -> ("output_L_Cue_laser_l1"=w493:i32)  [unwired: 11 in]
          n419 = call "BRig_arrTrig_L_Cue_event_l2.vi"() -> ("output_L_Cue_event_l2"=w492:i32)  [unwired: 11 in]
          n420 = call "BRig_arrTrig_L_Cue_laser_l2.vi"() -> ("output_L_Cue_laser_l2"=w488:i32)  [unwired: 11 in]
          n421 = call "BRig_arrTrig_L_Cue2_event_l1.vi"() -> ("output_L_Cue2_event_l1"=w489:i32)  [unwired: 11 in]
          n422 = call "BRig_arrTrig_L_Cue2_laser_l1.vi"() -> ("output_L_Cue2_laser_l1"=w490:i32)  [unwired: 11 in]
          n423 = call "BRig_arrTrig_L_Cue2_event_l2.vi"() -> ("output_L_Cue2_event_l2"=w491:i32)  [unwired: 11 in]
          n424 = call "BRig_arrTrig_L_Cue2_laser_l2.vi"() -> ("output_L_Cue2_laser_l2"=w495:i32)  [unwired: 11 in]
          n425 = Boolean To (0,1)(Boolean=w583) -> (0, 1=w587:i16)
          n426 = Boolean To (0,1)(Boolean=w580) -> (0, 1=w586:i16)
          n427 = Boolean To (0,1)(Boolean=w578) -> (0, 1=w584:i16)
          n428 = Boolean To (0,1)(Boolean=w576) -> (0, 1=w585:i16)
          n429 = Boolean To (0,1)(Boolean=w554) -> (0, 1=w565:i16)
          n430 = Boolean To (0,1)(Boolean=w553) -> (0, 1=w564:i16)
          n431 = Boolean To (0,1)(Boolean=w552) -> (0, 1=w562:i16)
          n432 = Boolean To (0,1)(Boolean=w551) -> (0, 1=w563:i16)
          n433 = Replace Array Subset(array=w589, new element #1=w583, index #1=w494, new element #2=w580, index #2=w493, new element #3=w578, index #3=w492, new element #4=w576, index #4=w488, new element #5=w554, index #5=w489, new element #6=w553, index #6=w490, new element #7=w552, index #7=w491, new element #8=w551, index #8=w495) -> (w588:bool[])
          n434 = To Unsigned Word Integer(number=w587) -> (unsigned 16bit integer=w582:u16)
          n435 = To Unsigned Word Integer(number=w586) -> (unsigned 16bit integer=w581:u16)
          n436 = To Unsigned Word Integer(number=w584) -> (unsigned 16bit integer=w579:u16)
          n437 = To Unsigned Word Integer(number=w585) -> (unsigned 16bit integer=w577:u16)
          n438 = To Unsigned Word Integer(number=w565) -> (unsigned 16bit integer=w560:u16)
          n439 = To Unsigned Word Integer(number=w564) -> (unsigned 16bit integer=w559:u16)
          n440 = To Unsigned Word Integer(number=w562) -> (unsigned 16bit integer=w558:u16)
          n441 = To Unsigned Word Integer(number=w563) -> (unsigned 16bit integer=w557:u16)
          n442 = Replace Array Subset(array=w546, new element #1=w582, index (row) #1=w561, index (col) #1=w483, new element #2=w581, index (row) #2=w561, index (col) #2=w482, new element #3=w579, index (row) #3=w561, index (col) #3=w481, new element #4=w577, index (row) #4=w561, index (col) #4=w480, new element #5=w560, index (row) #5=w561, index (col) #5=w479, new element #6=w559, index (row) #6=w561, index (col) #6=w478, new element #7=w558, index (row) #7=w561, index (col) #7=w477, new element #8=w557, index (row) #8=w561, index (col) #8=w476) -> (w575:u16[][])
        }
      }
    }
    frame False {
      w1018 = 0
      # "Record laser timing"
      # "Calculate laser timing"
      # "Total Time (Cue)"
      # "iTrial\nrelative"
      # "Total Time (Laser 2)"
      # "Total Time (Laser 1)"
      # "Current directionality, L or R?"
      # "Determine case for\ncalculating laser timing"
      # "2) Get relative iTrial"
      # "1) If Trial Start State = PostReward,\nThen check LC_Cue_nReward"
      # "laser2 active (Cue)?"
      # "laser1 active (Cue)?"
      # "1) If Trial Start State = PostReward,\nThen check LC_Cue_nReward\n\n2) Get relative iTrial"
      # "Gather variables"
      # "Last trial's\niReward\n(0 = not reward)"
      # "nTrials, current block"
      # "idx dataTrial"
      # "Total Time (Cue)"
      # "# PostReward Trials"
      # "Current directionality, L or R?"
      # "Total Time (Laser 2)"
      # "Total Time (Laser 1)"
      # "Calculate settings for Cue"
      # "Set laser settings for Cue and Cue2"
      # "iTrial\nrelative"
      # "laser timing case (Cue)"
      # "Trial start state\n0 (unknown)\n1 (first)\n2 (PreReward)\n3 (PostReward)"
      # "laser2 active?"
      # "laser1 active?"
      n443 = call "BRig_dataCurrent_iSpout.vi"() -> ("output_iSpout"=w1045:i32)  [unwired: 11 in]
      n444 = call "BRig_dataCurrent_LaserSwitch_l1.vi"() -> ("output_LaserSwitch_l1"=w1054:i32)  [unwired: 11 in]
      n445 = call "BRig_dataCurrent_LaserSwitch_l2.vi"() -> ("output_LaserSwitch_l2"=w1053:i32)  [unwired: 11 in]
      n446 = call "BRig_dataCurrent_iTrial.vi"() -> ("output_iTrial"=w1019:i32)  [unwired: 11 in]
      n447 = call "BRig_dataCurrent_T_Cue.vi"() -> ("output_T_Cue"=w1005:i32)  [unwired: 11 in]
      n448 = call "BRig_dataExp_L_Ttotal_l1.vi"() -> ("output_L_Ttotal_l1"=w1022:i32)  [unwired: 11 in]
      n449 = call "BRig_dataExp_L_Ttotal_l2.vi"() -> ("output_L_Ttotal_l2"=w1023:i32)  [unwired: 11 in]
      n450 = call "BRig_dataTrial_sTrial_start.vi"() -> ("output_sTrial_start"=w1050:i32)  [unwired: 11 in]
      n451 = call "BRig_dataTrial_iTrial_PostR.vi"() -> ("output_iTrial_PostR"=w1020:i32)  [unwired: 11 in]
      n452 = Index Array(array=w1029, index #1=w1045, index #2=w1054, index #3=w1053, index #4=w1019, index #5=w1005) -> (element #1=w1015:u16, element #2=w1052:u16, element #3=w1051:u16, element #4=w1009:u16, element #5=w1004:u16)
      n453 = Index Array(array=w1021, index #1=w1022, index #2=w1023) -> (element #1=w1017:u16, element #2=w1016:u16)
      n454 = Index Array(array=w1012, index (row) #1=w1018, index (col) #1=w1050, index (row) #2=w1018, index (col) #2=w1020) -> (element #1=w997:u16, element #2=w1008:u16)
      n455 = call "BRig_dataTrial_iReward.vi"() -> ("output_iReward"=w1013:i32)  [unwired: 11 in]
      n456 = Not Equal To 0?(x=w1052) -> (x != 0?=w1003:bool)
      n457 = Not Equal To 0?(x=w1051) -> (x != 0?=w1002:bool)
      n458 = Index Array(array=w1012, index (row)=1 ("disabled index (row)"), index (col)=w1013) -> (element=w1001:u16)
      n459 = case shown="3" w997 {
        tunnel: w1001 -> [_ _ w1099]
        tunnel: w1000 -> [_ _ w1100]
        tunnel: w1002 -> [_ w1092 w1094]
        tunnel: w1003 -> [_ w1093 w1095]
        tunnel: [w1091 w1093 w1098] -> w999
        tunnel: [w1091 w1092 w1097] -> w998
        frame 0 {
          w1091 = FALSE
        }
        frame 1, Default {
        }
        frame 3 {
          n460 = Boolean To (0,1)(Boolean=w1095) -> (0, 1=w1102:i16)
          n461 = Select(t=i16 2, s=w1094, f=i16 0) -> (s? t:f=w1103:i16)
          n462 = Compound Arithmetic op=ADD(w1102, w1103) -> (w1101:i16)
          n463 = case shown="3" w1101 {
            tunnel: w1100 -> [_ w1112 w1123 w1136]
            tunnel: w1099 -> [_ w1111 w1122 w1135]
            tunnel: [w1106 w1110 w1120 w1134] -> w1098
            tunnel: [w1106 w1109 w1121 w1133] -> w1097
            tunnel: FALSE -> [w1106 w1109 w1120 _]
            frame 0, Default {
            }
            frame 1 {
              n464 = call "BRig_dataLC_Cue_PostR_nRew1_l1.vi"() -> ("output_Cue_PostR_nRew1_l1"=w1107:i32)  [unwired: 11 in]
              n465 = call "BRig_dataLC_Cue_PostR_nRew2_l1.vi"() -> ("output_Cue_PostR_nRew2_l1"=w1108:i32)  [unwired: 11 in]
              n466 = Index Array(array=w1112, index #1=w1107, index #2=w1108) -> (element #1=w1114:u16, element #2=w1113:u16)
              n467 = Equal To 0?(x=w1114) -> (x = 0?=w1115:bool)
              n468 = Equal?(x=w1114, y=w1111) -> (x = y?=w1116:bool)
              n469 = Equal?(x=w1113, y=w1111) -> (x = y?=w1117:bool)
              n470 = Compound Arithmetic op=OR(w1115, w1116, w1117) -> (w1110:bool)
            }
            frame 2 {
              n471 = call "BRig_dataLC_Cue_PostR_nRew1_l2.vi"() -> ("output_Cue_PostR_nRew1_l2"=w1118:i32)  [unwired: 11 in]
              n472 = call "BRig_dataLC_Cue_PostR_nRew2_l2.vi"() -> ("output_Cue_PostR_nRew2_l2"=w1119:i32)  [unwired: 11 in]
              n473 = Index Array(array=w1123, index #1=w1118, index #2=w1119) -> (element #1=w1124:u16, element #2=w1125:u16)
              n474 = Equal To 0?(x=w1124) -> (x = 0?=w1127:bool)
              n475 = Equal?(x=w1124, y=w1122) -> (x = y?=w1126:bool)
              n476 = Equal?(x=w1125, y=w1122) -> (x = y?=w1128:bool)
              n477 = Compound Arithmetic op=OR(w1127, w1126, w1128) -> (w1121:bool)
            }
            frame 3 {
              n478 = call "BRig_dataLC_Cue_PostR_nRew1_l1.vi"() -> ("output_Cue_PostR_nRew1_l1"=w1129:i32)  [unwired: 11 in]
              n479 = call "BRig_dataLC_Cue_PostR_nRew2_l1.vi"() -> ("output_Cue_PostR_nRew2_l1"=w1130:i32)  [unwired: 11 in]
              n480 = call "BRig_dataLC_Cue_PostR_nRew1_l2.vi"() -> ("output_Cue_PostR_nRew1_l2"=w1131:i32)  [unwired: 11 in]
              n481 = call "BRig_dataLC_Cue_PostR_nRew2_l2.vi"() -> ("output_Cue_PostR_nRew2_l2"=w1132:i32)  [unwired: 11 in]
              n482 = Index Array(array=w1136, index #1=w1129, index #2=w1130, index #3=w1131, index #4=w1132) -> (element #1=w1140:u16, element #2=w1139:u16, element #3=w1137:u16, element #4=w1138:u16)
              n483 = Equal To 0?(x=w1140) -> (x = 0?=w1141:bool)
              n484 = Equal?(x=w1140, y=w1135) -> (x = y?=w1142:bool)
              n485 = Equal?(x=w1139, y=w1135) -> (x = y?=w1143:bool)
              n486 = Equal To 0?(x=w1137) -> (x = 0?=w1145:bool)
              n487 = Equal?(x=w1137, y=w1135) -> (x = y?=w1144:bool)
              n488 = Equal?(x=w1138, y=w1135) -> (x = y?=w1146:bool)
              n489 = Compound Arithmetic op=OR(w1141, w1142, w1143) -> (w1134:bool)
              n490 = Compound Arithmetic op=OR(w1145, w1144, w1146) -> (w1133:bool)
            }
          }
        }
      }
      n491 = case shown="1, Default" w997 {
        tunnel: [w1055 w1078 w1089] -> w996
        tunnel: [w1056 w1067 w1088] -> w995
        tunnel: [w1057 w1068 w1087] -> w994
        tunnel: [w1058 w1069 w1086] -> w993
        tunnel: [w1059 w1070 w1085] -> w992
        tunnel: [w1060 w1071 w1084] -> w991
        tunnel: [w1061 w1077 w1083] -> w990
        tunnel: [w1062 w1072 w1082] -> w989
        tunnel: [w1063 w1073 w1081] -> w988
        tunnel: [w1064 w1074 w1080] -> w987
        tunnel: [w1065 w1075 w1079] -> w986
        tunnel: [w1066 w1076 w1090] -> w985
        frame 1, Default {
          n492 = call "BRig_dataLC_Cue_First_OnOff_l1.vi"() -> ("output_Cue_First_OnOff"=w1055:i32)  [unwired: 11 in]
          n493 = call "BRig_dataLC_Cue_First_Block_l1.vi"() -> ("output_Cue_First_Block"=w1056:i32)  [unwired: 11 in]
          n494 = call "BRig_dataLC_Cue_First_Count_l1.vi"() -> ("output_Cue_First_Count"=w1057:i32)  [unwired: 11 in]
          n495 = call "BRig_dataLC_Cue_First_Prob_l1.vi"() -> ("output_Cue_First_Prob"=w1058:i32)  [unwired: 11 in]
          n496 = call "BRig_dataLC_Cue_First_Delay_l1.vi"() -> ("output_Cue_First_Delay"=w1059:i32)  [unwired: 11 in]
          n497 = call "BRig_dataLC_Cue_First_DelayOpt_l1.vi"() -> ("output_Cue_First_DelayOpt"=w1060:i32)  [unwired: 11 in]
          n498 = call "BRig_dataLC_Cue_First_OnOff_l2.vi"() -> ("output_Cue_First_OnOff_l2"=w1061:i32)  [unwired: 11 in]
          n499 = call "BRig_dataLC_Cue_First_Block_l2.vi"() -> ("output_Cue_First_Block_l2"=w1062:i32)  [unwired: 11 in]
          n500 = call "BRig_dataLC_Cue_First_Count_l2.vi"() -> ("output_Cue_First_Count_l2"=w1063:i32)  [unwired: 11 in]
          n501 = call "BRig_dataLC_Cue_First_Prob_l2.vi"() -> ("output_Cue_First_Prob_l2"=w1064:i32)  [unwired: 11 in]
          n502 = call "BRig_dataLC_Cue_First_Delay_l2.vi"() -> ("output_Cue_First_Delay_l2"=w1065:i32)  [unwired: 11 in]
          n503 = call "BRig_dataLC_Cue_First_DelayOpt_l2.vi"() -> ("output_Cue_First_DelayOpt_l2"=w1066:i32)  [unwired: 11 in]
        }
        frame 2 {
          n504 = call "BRig_dataLC_Cue_PreR_OnOff_l1.vi"() -> ("output_Cue_PreR_OnOff"=w1078:i32)  [unwired: 11 in]
          n505 = call "BRig_dataLC_Cue_PreR_Block_l1.vi"() -> ("output_Cue_PreR_Block"=w1067:i32)  [unwired: 11 in]
          n506 = call "BRig_dataLC_Cue_PreR_Count_l1.vi"() -> ("output_Cue_PreR_Count"=w1068:i32)  [unwired: 11 in]
          n507 = call "BRig_dataLC_Cue_PreR_Prob_l1.vi"() -> ("output_Cue_PreR_Prob"=w1069:i32)  [unwired: 11 in]
          n508 = call "BRig_dataLC_Cue_PreR_Delay_l1.vi"() -> ("output_Cue_PreR_Delay"=w1070:i32)  [unwired: 11 in]
          n509 = call "BRig_dataLC_Cue_PreR_DelayOpt_l1.vi"() -> ("output_Cue_PreR_DelayOpt"=w1071:i32)  [unwired: 11 in]
          n510 = call "BRig_dataLC_Cue_PreR_OnOff_l2.vi"() -> ("output_Cue_PreR_OnOff_l2"=w1077:i32)  [unwired: 11 in]
          n511 = call "BRig_dataLC_Cue_PreR_Block_l2.vi"() -> ("output_Cue_PreR_Block_l2"=w1072:i32)  [unwired: 11 in]
          n512 = call "BRig_dataLC_Cue_PreR_Count_l2.vi"() -> ("output_Cue_PreR_Count_l2"=w1073:i32)  [unwired: 11 in]
          n513 = call "BRig_dataLC_Cue_PreR_Prob_l2.vi"() -> ("output_Cue_PreR_Prob_l2"=w1074:i32)  [unwired: 11 in]
          n514 = call "BRig_dataLC_Cue_PreR_Delay_l2.vi"() -> ("output_Cue_PreR_Delay_l2"=w1075:i32)  [unwired: 11 in]
          n515 = call "BRig_dataLC_Cue_PreR_DelayOpt_l2.vi"() -> ("output_Cue_PreR_DelayOpt_l2"=w1076:i32)  [unwired: 11 in]
        }
        frame 3 {
          n516 = call "BRig_dataLC_Cue_PostR_OnOff_l1.vi"() -> ("output_Cue_PostR_OnOff"=w1089:i32)  [unwired: 11 in]
          n517 = call "BRig_dataLC_Cue_PostR_Block_l1.vi"() -> ("output_Cue_PostR_Block"=w1088:i32)  [unwired: 11 in]
          n518 = call "BRig_dataLC_Cue_PostR_Count_l1.vi"() -> ("output_Cue_PostR_Count"=w1087:i32)  [unwired: 11 in]
          n519 = call "BRig_dataLC_Cue_PostR_Prob_l1.vi"() -> ("output_Cue_PostR_Prob"=w1086:i32)  [unwired: 11 in]
          n520 = call "BRig_dataLC_Cue_PostR_Delay_l1.vi"() -> ("output_Cue_PostR_Delay"=w1085:i32)  [unwired: 11 in]
          n521 = call "BRig_dataLC_Cue_PostR_DelayOpt_l1.vi"() -> ("output_Cue_PostR_DelayOpt"=w1084:i32)  [unwired: 11 in]
          n522 = call "BRig_dataLC_Cue_PostR_OnOff_l2.vi"() -> ("output_Cue_PostR_OnOff_l2"=w1083:i32)  [unwired: 11 in]
          n523 = call "BRig_dataLC_Cue_PostR_Block_l2.vi"() -> ("output_Cue_PostR_Block_l2"=w1082:i32)  [unwired: 11 in]
          n524 = call "BRig_dataLC_Cue_PostR_Count_l2.vi"() -> ("output_Cue_PostR_Count_l2"=w1081:i32)  [unwired: 11 in]
          n525 = call "BRig_dataLC_Cue_PostR_Prob_l2.vi"() -> ("output_Cue_PostR_Prob_l2"=w1080:i32)  [unwired: 11 in]
          n526 = call "BRig_dataLC_Cue_PostR_Delay_l2.vi"() -> ("output_Cue_PostR_Delay_l2"=w1079:i32)  [unwired: 11 in]
          n527 = call "BRig_dataLC_Cue_PostR_DelayOpt_l2.vi"() -> ("output_Cue_PostR_DelayOpt_l2"=w1090:i32)  [unwired: 11 in]
        }
      }
      n528 = Less?(x=w997, y=u16 3) -> (x < y?=w1010:bool)
      n529 = Select(t=w1009, s=w1010, f=w1008) -> (s? t:f=w1007:u16)
      n530 = Boolean To (0,1)(Boolean=w999) -> (0, 1=w1047:i16)
      n531 = Select(t=i16 2, s=w998, f=i16 0) -> (s? t:f=w1048:i16)
      n532 = Add(x=w1047, y=w1048) -> (x+y=w1006:i16)
      n533 = case shown="3" w1006 {
        tunnel: w1000 -> [_ w1177 w1200 w1238]
        tunnel: w1015 -> [_ w1169 w1192 w1224]
        tunnel: w1004 -> [_ w1170 w1193 w1225]
        tunnel: w1007 -> [_ w1168 w1191 w1223]
        tunnel: [w1147 w1167 w1180 w1222] -> w1038
        tunnel: [w1147 w1166 w1180 w1221] -> w1035
        tunnel: [w1148 w1165 w1179 w1220] -> w1027
        tunnel: [w1148 w1164 w1179 w1219] -> w1026
        tunnel: [w1147 w1151 w1190 w1218] -> w1031
        tunnel: [w1148 w1150 w1189 w1217] -> w1025
        tunnel: [w1147 w1151 w1188 w1216] -> w1033
        tunnel: [w1148 w1150 w1187 w1215] -> w1024
        tunnel: w996 -> [_ w1163 _ w1214]
        tunnel: w995 -> [_ w1162 _ w1213]
        tunnel: w994 -> [_ w1161 _ w1212]
        tunnel: w993 -> [_ w1160 _ w1211]
        tunnel: w992 -> [_ w1159 _ w1210]
        tunnel: w991 -> [_ w1158 _ w1209]
        tunnel: w990 -> [_ w1157 w1186 w1208]
        tunnel: w989 -> [_ w1156 w1185 w1207]
        tunnel: w988 -> [_ w1155 w1184 w1206]
        tunnel: w987 -> [_ w1154 w1183 w1205]
        tunnel: w986 -> [_ w1153 w1182 w1204]
        tunnel: w985 -> [_ w1152 w1181 w1203]
        tunnel: w1017 -> [_ w1149 _ w1202]
        tunnel: w1016 -> [_ _ w1178 w1201]
        frame 0, Default {
          w1148 = u16 0
          w1147 = FALSE
          # "No active lasers"
        }
        frame 1 {
          w1150 = u16 0
          w1151 = FALSE
          # "laser1 is active"
          n534 = Index Array(array=w1177, index #1=w1163, index #2=w1162, index #3=w1161, index #4=w1160, index #5=w1159, index #6=w1158, index #7=w1157, index #8=w1156, index #9=w1155, index #10=w1154, index #11=w1153, index #12=w1152) -> (element #1=w1176:u16, element #2=w1175:u16, element #3=w1174:u16, element #4=w1173:u16, element #5=w1172:u16, element #6=w1171:u16)  [unwired: 6 out]
          n535 = call "BRig_RT__Case_Exp__State_initTrial__LC.vi"("input_L_OnOff"=w1176, "input_L_Block"=w1175, "input_L_Count"=w1174, "input_L_Prob"=w1173, "input_L_Tdelay"=w1172, "input_L_delayOpt"=w1171, "input_T_state"=w1170, "input_iSpout"=w1169, "input_iTrial_relative"=w1168, "input_L_T"=w1149) -> ("output_LC_Event"=w1167:bool, "output_LC_Laser"=w1166:bool, "output_L_Tstart"=w1165:u16, "output_L_Tend"=w1164:u16)  [unwired: 6 in]
        }
        frame 2 {
          w1179 = u16 0
          w1180 = FALSE
          # "laser2 is active"
          n536 = Index Array(array=w1200, index #1=w1186, index #2=w1185, index #3=w1184, index #4=w1183, index #5=w1182, index #6=w1181) -> (element #1=w1194:u16, element #2=w1195:u16, element #3=w1196:u16, element #4=w1197:u16, element #5=w1198:u16, element #6=w1199:u16)
          n537 = call "BRig_RT__Case_Exp__State_initTrial__LC.vi"("input_L_OnOff"=w1194, "input_L_Block"=w1195, "input_L_Count"=w1196, "input_L_Prob"=w1197, "input_L_Tdelay"=w1198, "input_L_delayOpt"=w1199, "input_T_state"=w1193, "input_iSpout"=w1192, "input_iTrial_relative"=w1191, "input_L_T"=w1178) -> ("output_LC_Event"=w1188:bool, "output_LC_Laser"=w1190:bool, "output_L_Tstart"=w1189:u16, "output_L_Tend"=w1187:u16)  [unwired: 6 in]
        }
        frame 3 {
          # "laser1 and laser2 are active"
          n538 = Index Array(array=w1238, index #1=w1214, index #2=w1213, index #3=w1212, index #4=w1211, index #5=w1210, index #6=w1209, index #7=w1208, index #8=w1207, index #9=w1206, index #10=w1205, index #11=w1204, index #12=w1203) -> (element #1=w1237:u16, element #2=w1236:u16, element #3=w1235:u16, element #4=w1234:u16, element #5=w1233:u16, element #6=w1232:u16, element #7=w1226:u16, element #8=w1227:u16, element #9=w1228:u16, element #10=w1229:u16, element #11=w1230:u16, element #12=w1231:u16)
          n539 = call "BRig_RT__Case_Exp__State_initTrial__LC.vi"("input_L_OnOff"=w1237, "input_L_Block"=w1236, "input_L_Count"=w1235, "input_L_Prob"=w1234, "input_L_Tdelay"=w1233, "input_L_delayOpt"=w1232, "input_T_state"=w1225, "input_iSpout"=w1224, "input_iTrial_relative"=w1223, "input_L_T"=w1202) -> ("output_LC_Event"=w1222:bool, "output_LC_Laser"=w1221:bool, "output_L_Tstart"=w1220:u16, "output_L_Tend"=w1219:u16)  [unwired: 6 in]
          n540 = call "BRig_RT__Case_Exp__State_initTrial__LC.vi"("input_L_OnOff"=w1226, "input_L_Block"=w1227, "input_L_Count"=w1228, "input_L_Prob"=w1229, "input_L_Tdelay"=w1230, "input_L_delayOpt"=w1231, "input_T_state"=w1225, "input_iSpout"=w1224, "input_iTrial_relative"=w1223, "input_L_T"=w1201) -> ("output_LC_Event"=w1216:bool, "output_LC_Laser"=w1218:bool, "output_L_Tstart"=w1217:u16, "output_L_Tend"=w1215:u16)  [unwired: 6 in]
        }
      }
      n541 = call "BRig_dataCurrent_L_Cue_T_start_l1.vi"() -> ("outputL_Cue_T_start_l1"=w984:i32)  [unwired: 11 in]
      n542 = call "BRig_dataCurrent_L_Cue_T_end_l1.vi"() -> ("output_L_Cue_T_end_l1"=w983:i32)  [unwired: 11 in]
      n543 = call "BRig_dataCurrent_L_Cue_T_start_l2.vi"() -> ("output_L_Cue_T_start_l2"=w982:i32)  [unwired: 11 in]
      n544 = call "BRig_dataCurrent_L_Cue_T_end_l2.vi"() -> ("output_L_Cue_T_end_l2"=w981:i32)  [unwired: 11 in]
      n545 = Replace Array Subset(array=w1029, new element #1=w1027, index #1=w984, new element #2=w1026, index #2=w983, new element #3=w1025, index #3=w982, new element #4=w1024, index #4=w981) -> (w1028:u16[])
      n546 = call "BRig_dataTrial_L_Cue_event_I_l1.vi"() -> ("output_L_Cue_event_I_l1"=w975:i32)  [unwired: 11 in]
      n547 = call "BRig_dataTrial_L_Cue_trig_I_l1.vi"() -> ("output_L_Cue_trig_I_l1"=w973:i32)  [unwired: 11 in]
      n548 = call "BRig_dataTrial_L_Cue_event_I_l2.vi"() -> ("output_L_Cue_event_I_l2"=w974:i32)  [unwired: 11 in]
      n549 = call "BRig_dataTrial_L_Cue_trig_I_l2.vi"() -> ("output_L_Cue_trig_I_l2"=w976:i32)  [unwired: 11 in]
      n550 = call "BRig_arrTrig_L_Cue_event_l1.vi"() -> ("output_L_Cue_event_l1"=w977:i32)  [unwired: 11 in]
      n551 = call "BRig_arrTrig_L_Cue_laser_l1.vi"() -> ("output_L_Cue_laser_l1"=w979:i32)  [unwired: 11 in]
      n552 = call "BRig_arrTrig_L_Cue_event_l2.vi"() -> ("output_L_Cue_event_l2"=w978:i32)  [unwired: 11 in]
      n553 = call "BRig_arrTrig_L_Cue_laser_l2.vi"() -> ("output_L_Cue_laser_l2"=w980:i32)  [unwired: 11 in]
      n554 = Boolean To (0,1)(Boolean=w1038) -> (0, 1=w1042:i16)
      n555 = Boolean To (0,1)(Boolean=w1035) -> (0, 1=w1041:i16)
      n556 = Boolean To (0,1)(Boolean=w1033) -> (0, 1=w1039:i16)
      n557 = Boolean To (0,1)(Boolean=w1031) -> (0, 1=w1040:i16)
      n558 = Replace Array Subset(array=w1044, new element #1=w1038, index #1=w977, new element #2=w1035, index #2=w979, new element #3=w1033, index #3=w978, new element #4=w1031, index #4=w980) -> (w1043:bool[])
      n559 = To Unsigned Word Integer(number=w1042) -> (unsigned 16bit integer=w1037:u16)
      n560 = To Unsigned Word Integer(number=w1041) -> (unsigned 16bit integer=w1036:u16)
      n561 = To Unsigned Word Integer(number=w1039) -> (unsigned 16bit integer=w1034:u16)
      n562 = To Unsigned Word Integer(number=w1040) -> (unsigned 16bit integer=w1032:u16)
      n563 = Replace Array Subset(array=w1012, new element #1=w1037, index (row) #1=w1018, index (col) #1=w975, new element #2=w1036, index (row) #2=w1018, index (col) #2=w973, new element #3=w1034, index (row) #3=w1018, index (col) #3=w974, new element #4=w1032, index (row) #4=w1018, index (col) #4=w976) -> (w1030:u16[][])
    }
  }
  "output_dataCurrent" <- w11
  "output_arrTrig" <- w14
  "output_dataTrial" <- w13
